vi "Martins HOT interface diag.vi"() -> ()   [LabVIEW 2012]
uses:
  Sub VIs/Trap cluster.ctl
  <vilib>/vision/Image Controls.llb/IMAQ Image.ctl
  Sub VIs/Get measurement coordinates.vi
  Sub VIs/Global variables.vi
  <vilib>/Utility/inputDevices.llb/closeKeyboard.vi
  <vilib>/Utility/inputDevices.llb/keyboardAcquire.vi
  <vilib>/Utility/file.llb/Write To Spreadsheet File (DBL).vi
  <vilib>/vision/driver/imaqhl.llb/IMAQ Grab Acquire.vi
  <vilib>/vision/driver/IMAQdx.llb/IMAQdx Grab.vi
  <vilib>/vision/driver/imaqll.llb/IMAQ Extract Buffer.vi
  Sub VIs/Get trap pos.vi
  <vilib>/Analysis/coordinate.llb/2D Cartesian Coordinate Shift.vi
  <vilib>/Analysis/coordinate.llb/2D Cartesian Coordinate Shift (Array).vi
  <vilib>/Analysis/coordinate.llb/2D Cartesian Coordinate Rotation.vi
  <vilib>/Analysis/coordinate.llb/2D Cartesian Coordinate Rotation (Scalar).vi
  <vilib>/vision/driver/NI_Vision_Acquisition_Software.lvlib
  <vilib>/vision/NI_Vision_Development_Module.lvlib
  <vilib>/Analysis/NI_AALPro.lvlib
panel:
  out "Using monitoring camera\nfor measurements":bool
  out "Measurement image":T1
  out "Monitoring image":T1
  in  "Apply Corrections":bool
  in  "View Licence":bool
  in  "ok":bool caption="Mark the center of \nthe spot using the \nzoom and the point\ntool, then click this \nbutton"
  in  "Stop program":bool
  in  "Updating trap cluster":bool
  out "Camera enabled":bool=TRUE
  out "SLM enabled":bool=TRUE
  in  "Hologram generation":cluster{"Method":i32, "Iterations":i32}={"Method"=1, "Iterations"=25} {"Method" items=["Lenses & Gratings (3D)", " Gerchberg-Saxton (3D)", "Gerchberg-Saxton FFT (2D)"]}
  in  "ROI":T2={"Global Rectangle"=[794, 414, 1159, 796], "Contours"=[{"Contour Type"=0, "ROI Type"=1, "Points"=[1158, 795]}, {"Contour Type"=0, "ROI Type"=1, "Points"=[898, 562]}, {"Contour Type"=0, "ROI Type"=1, "Points"=[794, 414]}]}
  out "Monitor image":T1(plugin-control)
  out "Waveform Graph":u32[](graph)
  out "max value":u32
  in  "reset":bool
  out "x/y":dbl
  in  "Outer bound":dbl=10.0
  in  "Inner bound":dbl=-10.0
  in  "stop \nsqueezing":bool
  in  "Squeeze":bool
  in  "Run meas calibration":bool
  in  "Display hologram\nand computed \nimage plane":bool
  in  "Run calibration":bool
  in  "Blank Button 2":bool
  in  "Blank Button":bool
  in  "subtract\nbackground":bool=TRUE
  in  "store \nbackground":bool
  in  "Coordinate mapping \n(Monitor to Measurement)":T3={"cZ"=1.0, "cY"=0.41527447, "cX"=-0.4158654, "sZ"=0.0, "sY"=-10.372314, "sX"=695.5264}
  in  "Transpose Measurement":bool
  out "Image\nsaturated":bool
  in  "Display ROIs":bool
  out "Lost Frames":u32=1
  in  "Display ROIs":bool
  out "Measurement image report":T4={"Mean Value"=58.96904, "Standard Variation"=5.129144, "Minimal Value"=35.0, "Maximal Value"=144.0, "Area (calibrated)"=65536.0, "Area (pixels)"=65536, "%"=100.0, "Calibration Valid"=TRUE} {"Mean Value" format="%.2f"; "%" format="%.2f"; "Area (calibrated)" format="%.2f"; "Maximal Value" format="%.2f"; "Minimal Value" format="%.2f"; "Standard Variation" format="%.2f"}
  in  "Save image path":path=path "E:/David/SLM characterization/Measured data/120420 - Trapping" caption="start path"
  in  "save image":bool
  in  "Edit trap cluster":bool
  in  "Display data":bool
  in  "Measure \nintensities":bool
  in  "Purge data":bool
  in  "ROI \nsize":dbl=24.0 min=2.0 step=2.0
  in  "Save data":bool
  in  "Record":bool
  in  "G":bool[](array[boolean])=[FALSE, FALSE, FALSE]
  out "Current trap pos":T5={"X (IMAQ)"=[1158.0, 898.0, 794.0], "Y (IMAQ)"=[795.0, 562.0, 414.0], "Z"=[0.0, 0.0, 0.0], "I"=[10.0, 10.0, 10.0], "Trap number"=[0, 1, 2], "ROI number"=[0, 1, 2], "Number of traps"=3, "Group"=[FALSE, FALSE, FALSE]}
  out "NI Vision error":errorcluster
  out "CUDA/SLM error":errorcluster
  in  "Cancel calibration":bool
  in  "Skip step if \ntimed out":bool
  in  "Display path":bool=TRUE
  out "Average step \ntime (ms)":dbl=14.596019900497513
  in  "Step \ntime \n(ms)":u32
  in  "Pause":bool
  in  "cancel path":bool
  out "Step \nskipped":bool
  in  "Path control":T6={"follow path"=FALSE, "Step \nlength"=0.2, "Arrive \nsimultaneously"=FALSE, "Synchronize traps"=FALSE, "Add current \npositions to path"=FALSE}
  in  "Create path":bool
  out "#":dbl[](array[numeric])=[0.0, 1.0, 2.0]
  in  "Group \nTraps":bool
  in  "Move \nHandle":bool
  in  "Coordinate mapping \n(IMAQ to SLM)":T3={"cZ"=1.0, "cY"=0.15274464, "cX"=0.15384616, "sZ"=-29.0, "sY"=-91.72315, "sX"=-108.5}
  in  "Transpose SLM":bool
  in  "I":dbl[](array[numeric])=[20.0, 20.0, 10.0]
  in  "Z":dbl[](array[numeric])=[0.0, 0.0, 0.0]
  # "Martin\nPersson 2011"
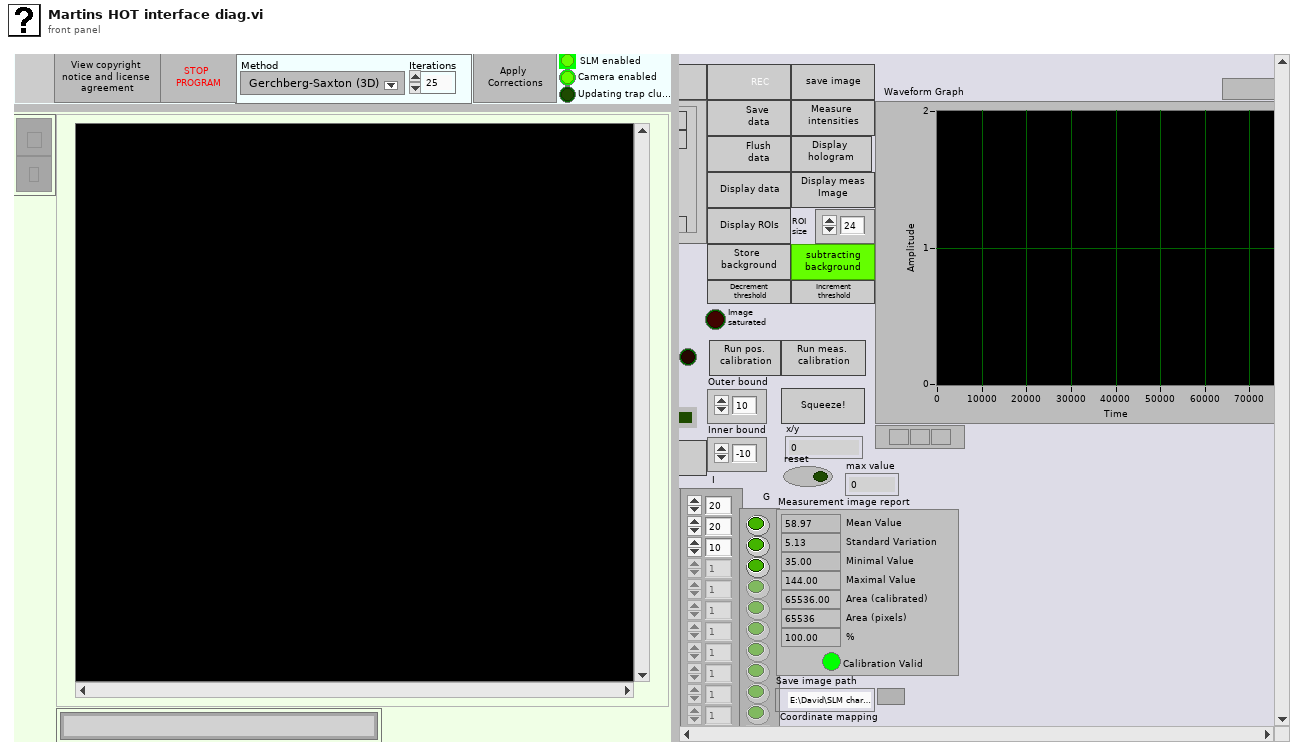
[diagram p1: front panel]
types:
  T1 = typedef "IMAQ Image.ctl" = refnum<image>
  T2 = cluster{"Global Rectangle":i32[], "Contours":cluster{"Contour Type":u32, "ROI Type":u32, "Points":i32[]}[]}
  T3 = cluster{"cZ":sgl, "cY":sgl, "cX":sgl, "sZ":sgl, "sY":sgl, "sX":sgl}
  T4 = cluster{"Mean Value":sgl, "Standard Variation":sgl, "Minimal Value":sgl, "Maximal Value":sgl, "Area (calibrated)":sgl, "Area (pixels)":u32, "%":sgl, "Calibration Valid":bool}
  T5 = typedef "Trap cluster.ctl" = cluster{"X (IMAQ)":sgl[], "Y (IMAQ)":sgl[], "Z":sgl[], "I":sgl[], "Trap number":i32[], "ROI number":i32[], "Number of traps":i32, "Group":bool[]}
  T6 = cluster{"follow path":bool, "Step \nlength":dbl, "Arrive \nsimultaneously":bool, "Synchronize traps":bool, "Add current \npositions to path":bool}
  T7 = cluster{"CentroidX":dbl[], "CentroidY":dbl[], "I":dbl[], "Acquired Buffer Number":u32}
  T8 = enum16{"IMAQ (Camera Link)", "IMAQ ring", "IMAQdx (firewire)", "No camera"}
  T9 = typedef "IMAQdx.ctl" = refnum<k21>
  T10 = cluster{"Camera type":enum16{"IMAQ (Camera Link)", "IMAQ ring", "IMAQdx (firewire)", "No camera"}, "IMAQ Session":refnum<k11>, "IMAQdx Session":T9, "Image":T1, "Image buffers":T1[], "Camera error":errorcluster}
  T11 = typedef "Image Type" = u32
  T12 = enum16{"Left Button", "Center Button", "Right Button", "Window Close"}
  T13 = typedef "ROI Descriptor" = cluster{"Global Rectangle":i32[], "Contours":cluster{"ID":enum32{"External", "Internal"}, "Type":u32, "Coordinates":i32[]}[]}
  T14 = enum16{"0", "1", "2", "3", "4", "5", "6", "7", "8", "9", "A", "B", "C", "D", "E", "F", "G", "H", "I", "J", "K", "L", "M", "N", "O", "P", "Q", "R", "S", "T", "U", "V", "W", "X", "Y", "Z", "F1", "F2", "F3", "F4", "F5", "F6", "F7", "F8", "F9", "F10", "F11", "F12", "F13", "F14", "F15", "ADD", "BACK", "BACKSLASH", "CAPITAL", "COMMA", "DECIMAL", "DELETE", "DIVIDE", "DOWN", "END", "EQUALS", "ESCAPE", "GRAVE (`)", "HOME", "INSERT", "LBRACKET", "LCONTROL", "LEFT", "L ALT", "LSHIFT", "LWIN", "MINUS", "MULTIPLY", "NEXT", "NUMLOCK", "NUMPAD_0", "NUMPAD_1", "NUMPAD_2", "NUMPAD_3", "NUMPAD_4", "NUMPAD_5", "NUMPAD_6", "NUMPAD_7", "NUMPAD_8", "NUMPAD_9", "PAUSE", "PERIOD", "PRIOR (PG UP)", "RBRACKET", "RCONTROL", "RETURN", "RIGHT", "R ALT", "RSHIFT", "RWIN", "SCROLL", "SEMICOLON", "SLASH", "SPACE", "SUBTRACT", "TAB", "UP", "ENTER (num pad)", "' (quote)"}[]
  T15 = cluster{"CentroidX":dbl[], "CentroidY":dbl[], "I":dbl[], "Acquired Buffer Number":u32}[]
  T16 = cluster{"Contour Type":u32, "ROI Type":u32, "Points":i32[]}[]
  T17 = cluster{"Contour Type":u32, "ROI Type":u32, "Points":i32[]}
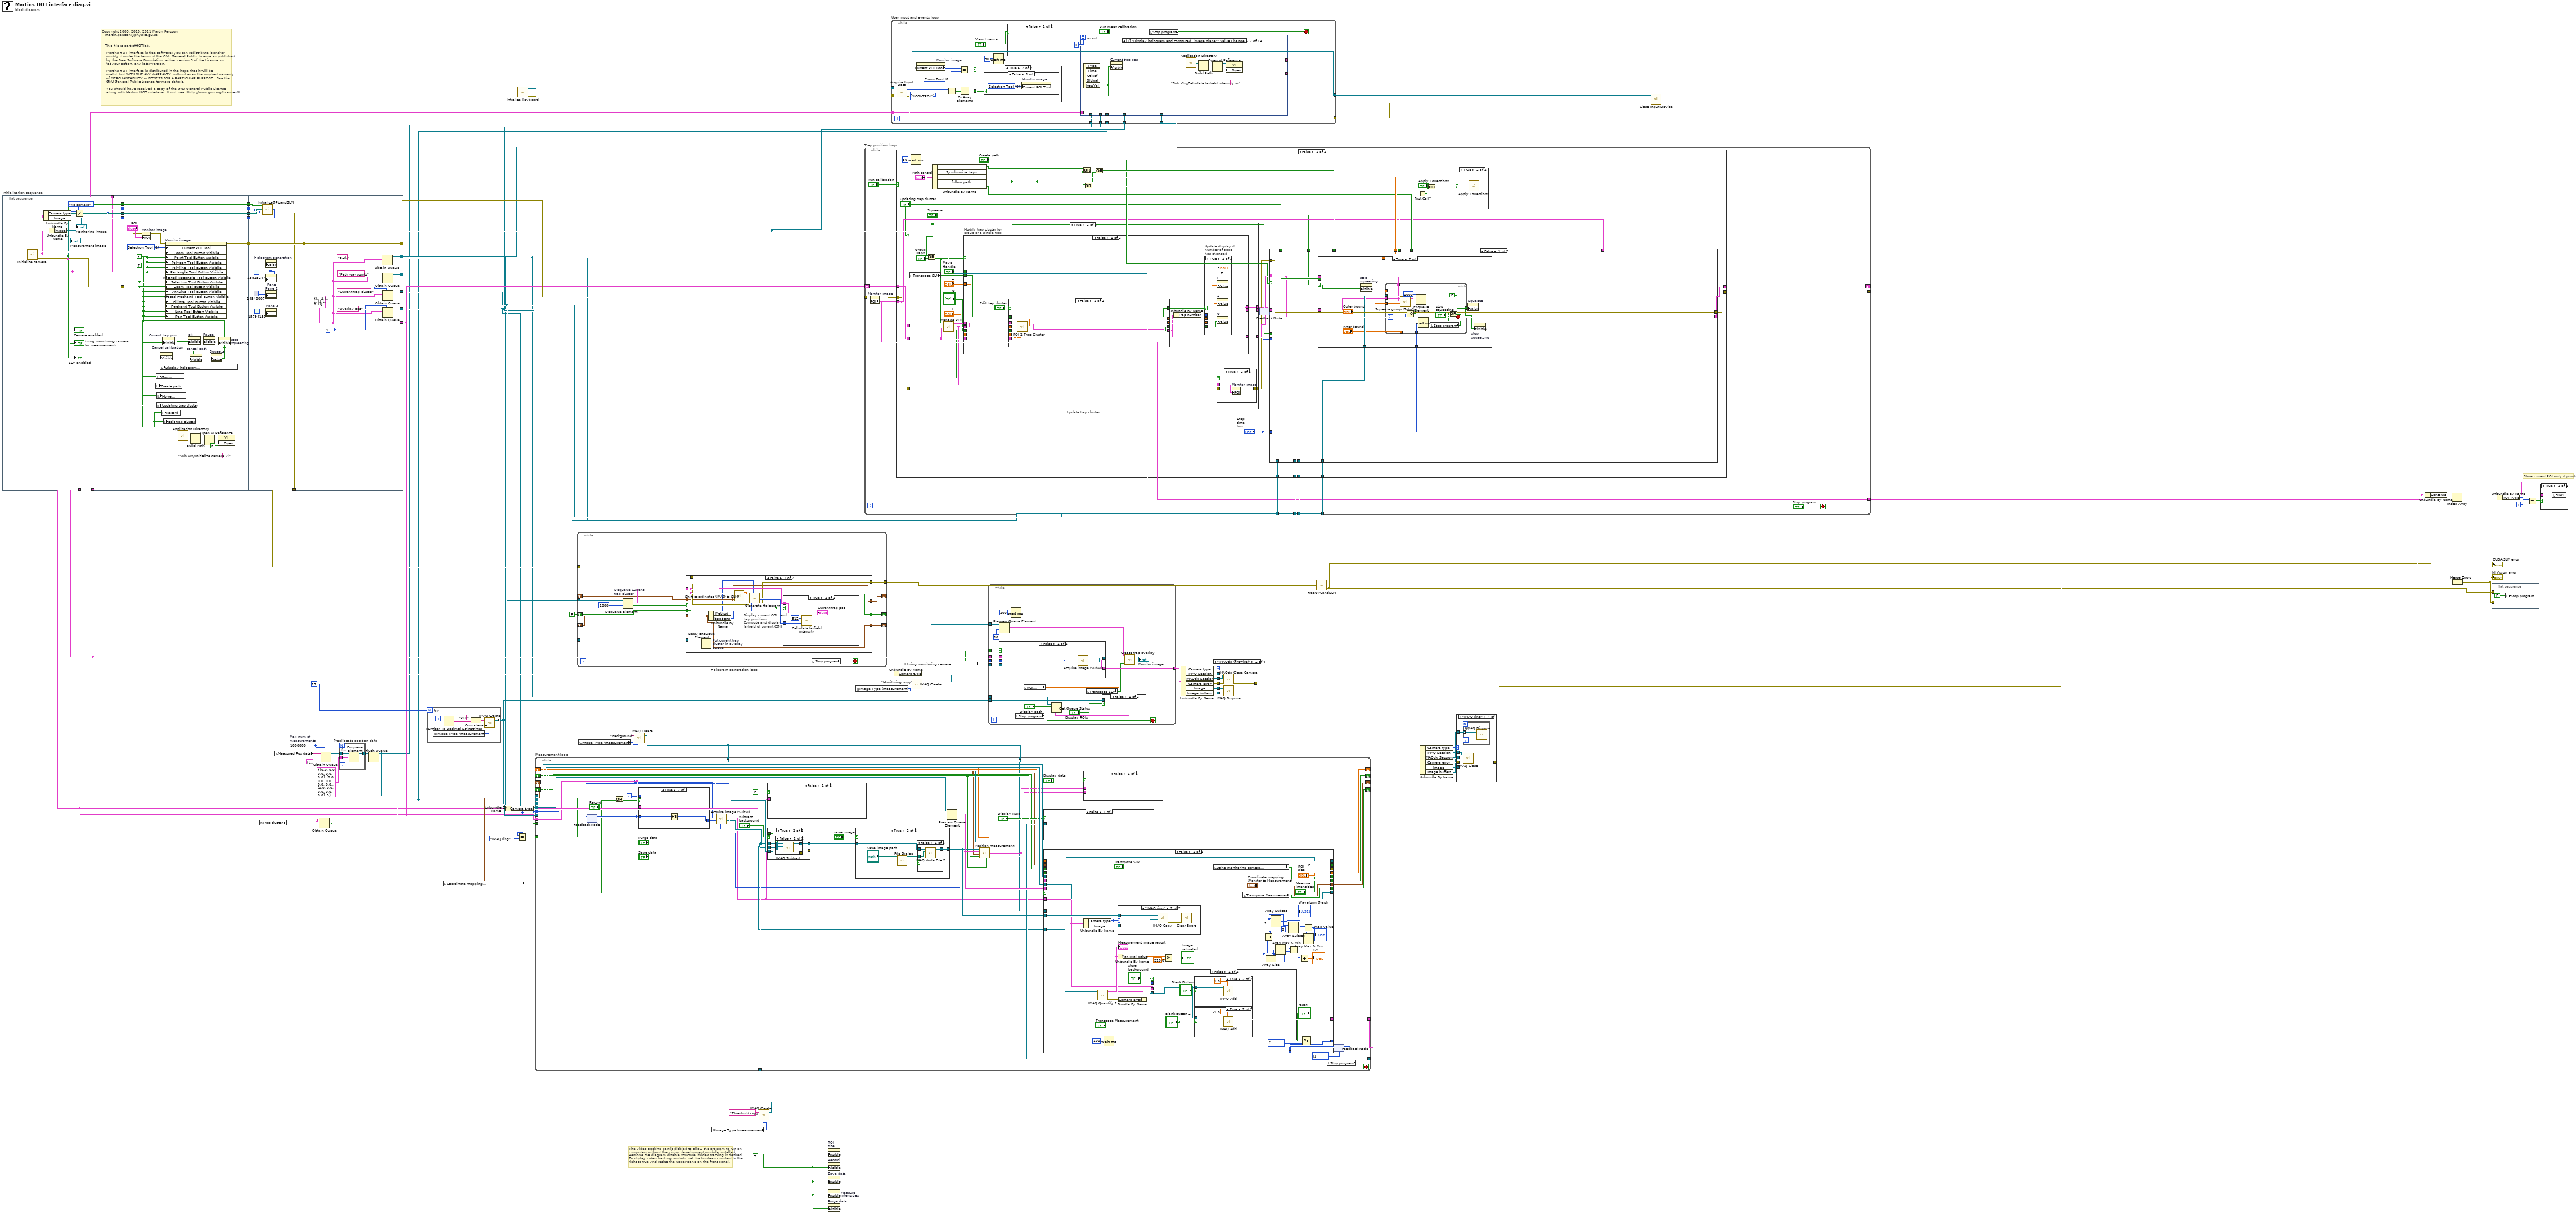
[diagram p0: block diagram]
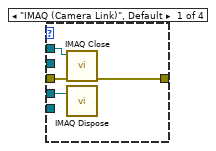
[diagram p2: hidden frame]
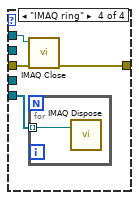
[diagram p4: hidden frame]
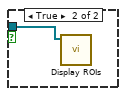
[diagram p5: hidden frame]
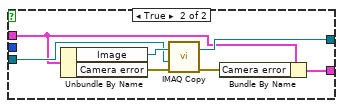
[diagram p6: hidden frame]
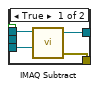
[diagram p8: hidden frame]
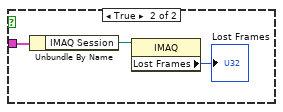
[diagram p9: hidden frame]
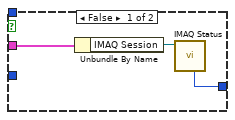
[diagram p10: hidden frame]
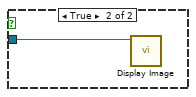
[diagram p11: hidden frame]
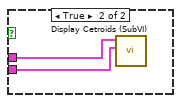
[diagram p12: hidden frame]
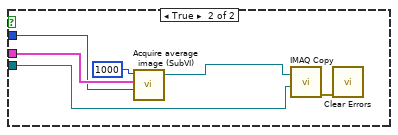
[diagram p17: hidden frame]
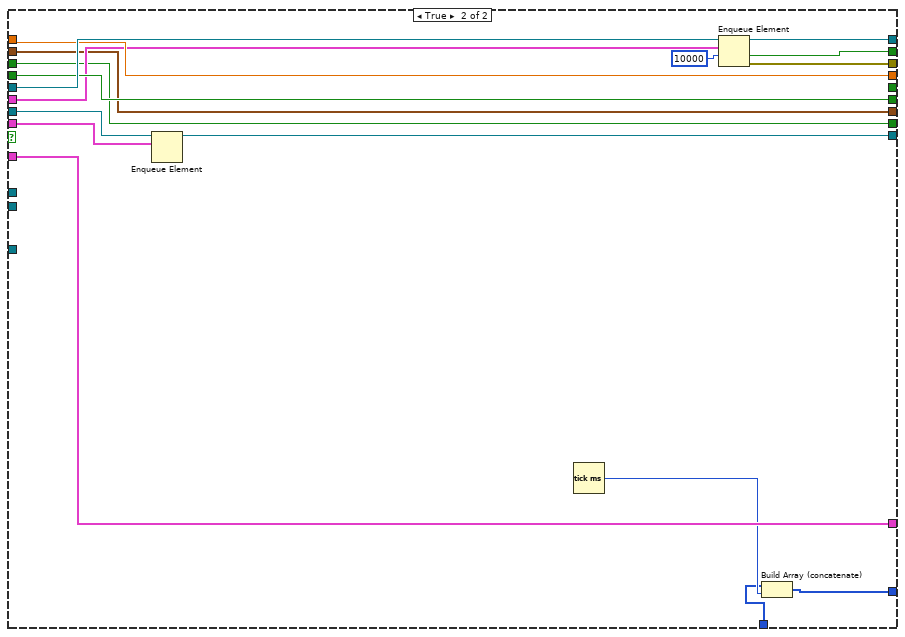
[diagram p19: hidden frame]
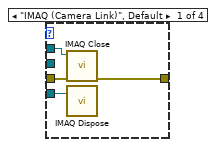
[diagram p20: hidden frame]
diagram:
  w1 = 1000000  # Max num of  measurements
  w77 = TRUE ("Visible")
  # "Copyright 2009, 2010, 2011 Martin Persson \n   martin.persson@physics.gu.se\n\n\n   This file is part ofHOTlab.\n\n    Martins HOT interface is free software: you can redistribute it and/or \n    modify it under the terms of the GNU General Public License as published \n    by the Free Software Foundation, either version 3 of the License, or\n    (at your option) any later version.\n\n    Martins HOT interface is distributed in the hope that it will be \n    useful, but WITHOUT ANY WARRANTY; without even the implied warranty\n    of MERCHANTABILITY or FITNESS FOR A PARTICULAR PURPOSE.  See the\n    GNU General Public License for more details.\n\n    You should have received a copy of the GNU General Public License\n    along with Martins HOT interface.  If not, see <http://www.gnu.org/licenses/>."
  # "Store current ROI only if points"
  # "The video tracking part is disbled to allow the program to run on\ncomputers without the vision development module installed. \nRemove the diagram disable structure ifvideo tracking is desired. \nTo diplay video tracking controls, set the boolean constant to the \nright to true And resize the upper pane on the front panel."
  n1 = flat-sequence "Initialization sequence" {
    tunnel: [w88] -> w63
    tunnel: [w92] -> w62
    tunnel: [w91] -> w61
    tunnel: [w90] -> w60
    tunnel: [w89] -> w59
    tunnel: [w83] -> w37
    tunnel: [w81] -> w9
    tunnel: [w81] -> w47
    tunnel: w63 -> [w105]
    tunnel: w62 -> [w103]
    tunnel: w61 -> [w108]
    tunnel: w60 -> [w107]
    tunnel: w59 -> [w106]
    tunnel: [w105] -> w55
    tunnel: [w100] -> w54
    tunnel: [w108] -> w52
    tunnel: [w107] -> w51
    tunnel: [w106] -> w50
    tunnel: w55 -> [w114]
    tunnel: w54 -> [w117]
    tunnel: [w117] -> w53
    tunnel: w52 -> [w115]
    tunnel: w51 -> [w116]
    tunnel: w50 -> [w113]
    tunnel: [w112] -> w49
    tunnel: [w128] -> w58
    tunnel: w53 -> [w128]
    tunnel: [w126] -> w24
    tunnel: [w124] -> w57
    tunnel: [w122] -> w48
    tunnel: [w121] -> w25
    tunnel: [w118] -> w56
    frame #0 {
      n2 = call "Initialize camera.vi"() -> ("Use monitoring camera\nfor measurements"=→"Using monitoring camera\nfor measurements":bool, "Vision error out"=w92:errorcluster, "CUDA device ID"=w90:i32, "TrueFrame out"=w91:i32, "Measurement camera cluster"=w81:T10, "LUT path out"=w89:path, "SLM enabled"=w88:bool, "Monitoring camera cluster"=w83:T10)  [unwired: 3 in]
      "SLM enabled" <- w88
      n3 = Unbundle By Name(w83) -> ("Camera type"=w85:T8, "Image"=→"Monitoring image":T1)
      n4 = Unbundle By Name(w81) -> ("Image"=→"Measurement image":T1)
      n5 = Not Equal?(x=w85, y=T8."No camera") -> (x != y?=→"Camera enabled":bool)
    }
    frame #1 {
      w99 = TRUE ("ROI Tool Buttons Visibile:Zoom Tool Button Visible")
      w98 = FALSE ("ROI Tool Buttons Visibile:Zoom Tool Button Visible")
      w102 = u32 0 items=["Zoom Tool"=8, "Selection Tool"=0, "Pan Tool"=9, "Point Tool"=1, "Line Tool"=2, "Rectangle Tool"=3, "Rotated Rectangle Tool"=12, "Polyline Tool"=10, "Polygon Tool"=5, "Freehand Tool"=11, "Closed Freehand Tool"=6, "Ellipse Tool"=4, "Annulus Tool"=7] ("Current ROI Tool")
      n6 = property on="Monitor image" class="ImageControl"(error in=w103, "ROI"="ROI") -> (error out=w101:errorcluster)  [unwired: 1 in, 1 out]
      n7 = local write "Create path"(w98) -> ()
      n8 = local write "Group \nTraps"(w98) -> ()
      n9 = local write "Move \nHandle"(w98) -> ()
      n10 = local write "Updating trap cluster"(w99) -> ()
      n11 = property on="Cancel calibration" class="Bool"("Visible"=w98) -> ()  [unwired: 2 in, 2 out]
      n12 = local write "Display hologram\nand computed \nimage plane"(w98) -> ()
      n13 = local write "Record"(w98) -> ()
      n14 = property on="Current trap pos" class="Clust (strict)"("Visible"=w98) -> ()  [unwired: 2 in, 2 out]
      n15 = local write "Edit trap cluster"(w98) -> ()
      n16 = property on="Monitor image" class="ImageControl"(error in=w101, "Current ROI Tool"=w102, "Zoom Tool Button Visibile"=w98, "Point Tool Button Visibile"=w98, "Polygon Tool Button Visibile"=w98, "Polyline Tool Button Visibile"=w98, "Rectangle Tool Button Visibile"=w98, "Rotated Rectangle Tool Button Visibile"=w98, "Selection Tool Button Visibile"=w99, "Zoom Tool Button Visibile"=w99, "Annulus Tool Button Visibile"=w98, "Closed Freehand Tool Button Visibile"=w98, "Ellipse Tool Button Visibile"=w98, "Freehand Tool Button Visibile"=w98, "Line Tool Button Visibile"=w98, "Pan Tool Button Visibile"=w98) -> (error out=w100:errorcluster)  [unwired: 1 in, 1 out]
      n17 = call <vilib>:"Application Directory.vi"() -> ("Application Directory"=w94:path)
      n18 = property on="ok" class="Bool"("Visible"=w98) -> ()  [unwired: 2 in, 2 out]
      n19 = property on="cancel path" class="Bool"("Visible"=w98) -> ()  [unwired: 2 in, 2 out]
      n20 = Build Path(base path=w94, name or relative path="Sub VIs\\Initialize camera.vi") -> (appended path=w97:path)
      n21 = property on="Pause" class="Bool (strict)"("Visible"=w98) -> ()  [unwired: 2 in, 2 out]
      n22 = Open VI Reference(vi path=w97) -> (vi reference=w96:refnum<vi>)  [unwired: 5 in, 1 out]
      n23 = property on="Squeeze" class="Bool (strict)"("Value"=w98) -> ()  [unwired: 2 in, 2 out]
      n24 = property class="VI"(reference=w96, "Front Panel.Open"=FALSE ("Front Panel Window:Open")) -> ()  [unwired: 1 in, 2 out]
      n25 = property on="stop \nsqueezing" class="Bool"("Visible"=w98) -> ()  [unwired: 2 in, 2 out]
    }
    frame #2 {
      w109 = u32 15925247 ("Pane Color")
      n26 = call "InitializeGPUandSLM.vi"("TrueFrame"=w115, "deviceId"=w116, "Path to LUT file"=w113, "SLM enabled"=w114) -> ("CUDA/SLM error"=w112:errorcluster)  [unwired: 1 out]
      n27 = property on="Hologram generation" class="Clust (strict)"("Color"=w109) -> ()  [unwired: 2 in, 2 out]
      n28 = property on="Pane" class="Pane"("PaneColor"=w109) -> ()  [unwired: 2 in, 2 out]
      n29 = property on="Pane 2" class="Pane"("PaneColor"=u32 14540007 ("Pane Color")) -> ()  [unwired: 2 in, 2 out]
      n30 = property on="Pane 3" class="Pane"("PaneColor"=u32 15794150 ("Pane Color")) -> ()  [unwired: 2 in, 2 out]
    }
    frame #3 {
      w118 = T5 {"X (IMAQ)"=[], "Y (IMAQ)"=[], "Z"=[], "I"=[], "Trap number"=[], "ROI number"=[], "Number of traps"=0, "Group"=[]} ("output cluster 2")
      w119 = 1 ("max queue size (-1, unlimited)")
      n31 = Obtain Queue(name (unnamed)="Path", element data type=w118) -> (queue out=w126:refnum<queue>)  [unwired: 3 in, 2 out]
      n32 = Obtain Queue(name (unnamed)="Path waypoints", element data type=w118) -> (queue out=w124:refnum<queue>)  [unwired: 3 in, 2 out]
      n33 = Obtain Queue(max queue size (-1, unlimited)=w119, name (unnamed)="Current trap cluster", element data type=w118) -> (queue out=w122:refnum<queue>)  [unwired: 2 in, 2 out]
      n34 = Obtain Queue(max queue size (-1, unlimited)=w119, name (unnamed)="Overlay pos", element data type=w118) -> (queue out=w121:refnum<queue>)  [unwired: 2 in, 2 out]
    }
  }
  n35 = global read "Global variables.vi" "Trap cluster"() -> (w13:string)
  n36 = global read "Global variables.vi" "Measured Pos data"() -> (w12:string)
  n37 = Obtain Queue(name (unnamed)=w13, element data type=w56) -> (queue out=w10:refnum<queue>, created new?=w11:bool)  [unwired: 3 in, 1 out]
  n38 = Obtain Queue(max queue size (-1, unlimited)=w1, name (unnamed)=w12, element data type=T7 {"CentroidX"=[], "CentroidY"=[], "I"=[], "Acquired Buffer Number"=0} ("Position data out")) -> (queue out=w5:refnum<queue>)  [unwired: 2 in, 2 out]
  n39 = for "Preallocate position data" {
    N: w1 -> [_]
    tunnel: w5 -> [w131]
    tunnel: T7 {"CentroidX"=[0.0, 0.0, 0.0, 0.0, 0.0], "CentroidY"=[0.0, 0.0, 0.0, 0.0, 0.0], "I"=[0.0, 0.0, 0.0, 0.0, 0.0], "Acquired Buffer Number"=5} ("Position data out") -> [w130]
    tunnel: [w129] -> w3
    n40 = Enqueue Element(queue=w131, element=w130) -> (queue out=w129:refnum<queue>)  [unwired: 2 in, 2 out]
  }
  n41 = Flush Queue(queue=w3) -> (queue out=w2:refnum<queue>)  [unwired: 1 in, 2 out]
  n42 = for {
    N: 25 -> [_]
    tunnel: [w137] -> w23 mode=indexing
    i -> [w134]
    n43 = global read "Global variables.vi" "Image Type (measurement)"() -> (w132:T11)
    n44 = Number To Decimal String(number=w134) -> (decimal integer string=w133:string)  [unwired: 1 in]
    n45 = Concatenate Strings("ROI" ("Image Name"), w133) -> (w135:string)
    n46 = call "IMAQ Create"("Image Name"=w135, "Image Type"=w132) -> ("New Image"=w137:T1)  [unwired: 3 in, 1 out]
  }
  n47 = local read "Coordinate mapping \n(Monitor to Measurement)"() -> (w18:T3)
  n48 = Unbundle By Name(w9) -> ("Camera type"=w7:T8)
  n49 = Not Equal?(x=w7, y=T8."IMAQ ring") -> (x != y?=w8:bool)
  n50 = call <vilib>:"Intialize Keyboard.vi"() -> ("error out"=w65:errorcluster, "device ID"=w79:refnum<k1>)  [unwired: 1 in, 9 out]
  n51 = while "Hologram generation loop" {
    tunnel: w48 -> [w149]
    tunnel: w25 -> [w147]
    tunnel: w49 -> [w146]
    tunnel: [w145] -> w46
    shift-right: [w144] -> _
    shift-left: _ -> [w143]
    shift-right: [w142] -> _
    shift-left: _ -> [w141]
    shift-right: [w140] -> _
    shift-left: FALSE ("Display hologram\nand computed \nimage plane") -> [w139]
    stop <- w150 stop-if-true
    n52 = Dequeue Element "Dequeue Current \ntrap cluster"(queue=w149, timeout in ms (-1)=1000) -> (element=w148:T5, timed out?=w138:bool)  [unwired: 1 in, 2 out]
    n53 = case shown="False" w138 {
      tunnel: w143 -> [w156 _]
      tunnel: w148 -> [w160 _]
      tunnel: w147 -> [w159 _]
      tunnel: w146 -> [w158 w172]
      tunnel: [w157 w172] -> w145
      tunnel: [w156 "Coordinate mapping \n(IMAQ to SLM)"] -> w144
      tunnel: [w153 "Hologram generation"] -> w142
      tunnel: w141 -> [w153 _]
      tunnel: [w152 "Display hologram\nand computed \nimage plane"] -> w140
      tunnel: w139 -> [w152 _]
      frame False {
        n54 = Lossy Enqueue Element "Put current trap \ncluster in overlay \nqueue"(queue=w159, element=w160) -> ()  [unwired: 1 in, 4 out]
        n55 = Unbundle By Name(w153) -> ("Method"=w155:i32, "Iterations"=w154:i32)
        n56 = call "Shift coordinates (IMAQ to SLM).vi"("Trap cluster"=w160, "Coordinate mapping \n(IMAQ to SLM)"=w156) -> ("X (SLM)"=w161:sgl[], "Y (SLM)"=w164:sgl[], "Intensities"=w162:sgl[], "Z (SLM)"=w163:sgl[])  [unwired: 1 in, 1 out]
        n57 = call "Generate Hologram.vi"("x"=w161, "y"=w164, "z"=w163, "spot_intensities"=w162, "CUDA/SLM error in"=w158, "N_iterations"=w154, "method"=w155) -> ("CGH out"=w165:u8[][], "CUDA/SLM error out"=w157:errorcluster)  [unwired: 17 in, 2 out]
        n58 = case "Display current CGH and trap positions.\nCompute and display farfield of current CGH" shown="True" w152 {
          tunnel: w165 -> [_ w168]
          tunnel: w160 -> [_ w167]
          frame False {
          }
          frame True {
            n59 = call "Calculate farfield intensity.vi"("h_pSLM"=w168, "SLMsize"=512 ("Numeric")) -> ()  [unwired: 1 out]
            "Current trap pos" <- w167
          }
        }
      }
      frame True {
      }
    }
    n60 = local read "Stop program"() -> (w150:bool)
  }
  n61 = global read "Global variables.vi" "Image Type (measurement)"() -> (w16:T11)
  n62 = call "IMAQ Create"("Image Name"="Background", "Image Type"=w16) -> ("New Image"=w14:T1)  [unwired: 3 in, 1 out]
  n63 = global read "Global variables.vi" "Image Type (measurement)"() -> (w20:T11)
  n64 = call "IMAQ Create"("Image Name"="Threshold copy", "Image Type"=w20) -> ("New Image"=w22:T1)  [unwired: 3 in, 1 out]
  n65 = while "Measurement loop" {
    tunnel: w23 -> [w203]
    tunnel: w2 -> [w212]
    shift-right: [w211] -> _
    shift-left: _ -> [w201]
    tunnel: w10 -> [w210]
    shift-right: [w209] -> _
    shift-left: _ -> [w202]
    tunnel: [w204] -> _
    tunnel: w9 -> [w194]
    tunnel: w25 -> [w206]
    tunnel: w24 -> [_]
    tunnel: [w207] -> w40
    tunnel: w7 -> [w180]
    tunnel: w22 -> [w184]
    shift-right: [w197] -> _
    shift-left: w18 -> [w196]
    shift-right: [w190] -> _
    shift-left: _ -> [w189]
    tunnel: w14 -> [w188]
    tunnel: w14 -> [w186]
    tunnel: w11 -> [_]
    tunnel: w8 -> [w178]
    i -> [w192]
    stop <- w213 stop-if-true
    n66 = feedback #1() -> (w182:u32)  [unwired: 1 in]
    n67 = Or(x=w178, y="Record") -> (x .or. y?=w179:bool)
    n68 = case shown="True" w179 {
      tunnel: w194 -> [w235 _]
      tunnel: [w233 w236] -> w193
      tunnel: w192 -> [_ _]
      tunnel: w182 -> [_ w237]
      frame False {
        n69 = Unbundle By Name(w235) -> ("IMAQ Session"=w234:refnum<k11>)
        n70 = call <vilib>:"IMAQ Status.vi"("IMAQ Session In"=w234) -> ("Last Valid Buffer Number"=w233:i32)  [unwired: 6 in, 4 out]
      }
      frame True {
        n71 = Increment(x=w237) -> (x+1=w236:u32)
      }
    }
    n72 = call "Acquire image (SubVI).vi"("Buffer number"=w193, "Camera type"=w180, "Measurement camera \ncluster in"=w194) -> ("Image Out"=w181:T1, "Measurement camera cluster out"=w177:T10, "Buffer Number Out"=w183:u32)  [unwired: 6 in]
    n73 = feedback-in #1(w183) -> ()
    n74 = case shown="False" FALSE {
      tunnel: w177 -> [_ w230]
      frame False {
      }
      frame True {
        n75 = Unbundle By Name(w230) -> ("IMAQ Session"=w232:refnum<k11>)
        n76 = property class="IMAQ"(reference=w232) -> ("Lost Frames"=→"Lost Frames":u32)  [unwired: 1 in, 2 out]
      }
    }
    n77 = case shown="True" "subtract\nbackground" {
      tunnel: [w214 w220] -> w187
      tunnel: w181 -> [w214 w219]
      tunnel: w186 -> [_ w218]
      tunnel: [_ w217] -> _
      tunnel: w184 -> [_ w215]
      tunnel: "Record" -> [_ w216]
      frame False {
      }
      frame True {
        n78 = case shown="False" w216 {
          tunnel: [w224 w229] -> w220
          tunnel: w219 -> [w223 w228]
          tunnel: w218 -> [w222 w227]
          tunnel: [w221 w226] -> w217
          tunnel: w215 -> [_ w225]
          frame True {
            n79 = call "IMAQ Subtract"("Image Src A"=w223, "Image Src B"=w222) -> ("Image Dst Out"=w224:T1, "error out"=w221:errorcluster)  [unwired: 5 in]
          }
          frame False {
            n80 = call "IMAQ Subtract"("Image Src A"=w228, "Image Dst"=w225, "Image Src B"=w227) -> ("Image Dst Out"=w229:T1, "error out"=w226:errorcluster)  [unwired: 4 in]
          }
        }
      }
    }
    n81 = case shown="True" "save image" {
      tunnel: w187 -> [w241 w246]
      tunnel: [w241 w245] -> w204
      frame False {
      }
      frame True {
        n82 = call "File Dialog"("start path"="Save image path") -> ("selected path"=w244:path, "cancelled"=w243:bool)  [unwired: 11 in, 2 out]
        n83 = case shown="False" w243 {
          tunnel: w246 -> [w249 w250]
          tunnel: [w248 w250] -> w245
          tunnel: w244 -> [w247 _]
          frame False {
            n84 = call-poly "IMAQ Write File 2"("File Path"=w247, "Image"=w249) -> ("Image Out (duplicate)"=w248:T1)  [unwired: 8 in, 1 out]
          }
          frame True {
          }
        }
      }
    }
    n85 = Preview Queue Element(queue=w206) -> (element=w205:T5)  [unwired: 2 in, 3 out]
    n86 = call "Position measurement.vi"("Measure \nintensities"=w202, "ROI size"=w201, "Acquired Buffer Number"=w182, "Switch xy"=w189, "Coordinate mapping \n(Monitor to Measurement)"=w196, "ROIs"=w203, "Trap positions"=w205, "Image"=w204) -> ("Target coordinates"=w195:cluster{"X target":sgl[], "Y target":sgl[]}, "Position data out"=w199:T7)  [unwired: 1 in]
    n87 = case shown="False" "Display ROIs" {
      tunnel: w204 -> [_ w238]
      frame False {
      }
      frame True {
        n88 = call "Display Image.vi"("Image 2"=w238) -> ()  [unwired: 11 in]
      }
    }
    n89 = case shown="False" "Display data" {
      tunnel: w199 -> [_ w240]
      tunnel: w195 -> [_ w239]
      frame False {
      }
      frame True {
        n90 = call "Display Cetroids (SubVI).vi"("Target coordinates"=w239, "Measurement data"=w240) -> ()  [unwired: 7 in, 3 out]
      }
    }
    n91 = local read "Stop program"() -> (w213:bool)
    n92 = feedback #2(u32[] []) -> (w175:u32[])
    n93 = case shown="False" "Record" {
      tunnel: w212 -> [w288 w321]
      tunnel: [w288 w320] -> _
      tunnel: [_ w319] -> _
      tunnel: ["ROI \nsize" w318] -> w211
      tunnel: w201 -> [_ w318]
      tunnel: w210 -> [w287 w317]
      tunnel: [w287 w316] -> _
      tunnel: ["Measure \nintensities" w315] -> w209
      tunnel: w202 -> [_ w315]
      tunnel: [FALSE ("timed out?") w313] -> _
      tunnel: w204 -> [w271 _]
      tunnel: w177 -> [w269 w312]
      tunnel: [w281 w312] -> w207
      tunnel: w205 -> [_ w311]
      tunnel: w199 -> [_ w310]
      tunnel: ["Coordinate mapping \n(Monitor to Measurement)" w309] -> w197
      tunnel: w196 -> [_ w309]
      tunnel: [w275 _] -> _
      tunnel: [w273 w308] -> w190
      tunnel: w189 -> [_ w308]
      tunnel: w188 -> [w270 _]
      tunnel: w181 -> [w267 _]
      tunnel: [w266 w307] -> w176
      tunnel: w175 -> [w255 w305]
      frame False {
        n94 = Unbundle By Name(w269) -> ("Camera type"=w268:T8, "Image"=w274:T1)
        n95 = call "IMAQ Quantify 2"("Image"=w267) -> ("error out"=w282:errorcluster, "Global Report"=w280:T4)  [unwired: 8 in, 1 out]
        "Measurement image report" <- w280
        n96 = Wait (ms)(milliseconds to wait=u32 100) -> ()  [unwired: 1 out]
        n97 = case shown="\"IMAQ ring\"" w268 {
          tunnel: w271 -> [_ w304]
          tunnel: w274 -> [_ w303]
          frame "IMAQ (Camera Link)", Default {
          }
          frame "IMAQ ring" {
            n98 = call "IMAQ Copy"("Image Dst"=w303, "Image Src"=w304) -> ("error out"=w302:errorcluster)  [unwired: 4 in, 1 out]
            n99 = call <vilib>:"Clear Errors.vi"("error in (no error)"=w302) -> ()  [unwired: 6 in, 1 out]
          }
        }
        n100 = Unbundle By Name(w280) -> ("Maximal Value"=w279:sgl)
        n101 = Bundle By Name(cluster=w269, "Camera error"=w282) -> (w281:T10)
        n102 = case shown="False" "store \nbackground" {
          tunnel: w270 -> [w291 w300]
          tunnel: w269 -> [_ w299]
          tunnel: w268 -> [_ w298]
          frame False {
            n103 = case shown="True" "Blank Button" {
              tunnel: w291 -> [_ w295]
              frame False {
              }
              frame True {
                n104 = call "IMAQ Add"("Image Src A"=w295, "Constant"=sgl 1.0) -> ()  [unwired: 5 in, 2 out]
              }
            }
            n105 = case shown="True" "Blank Button 2" {
              tunnel: w291 -> [_ w293]
              frame False {
              }
              frame True {
                n106 = call "IMAQ Add"("Image Src A"=w293, "Constant"=sgl -1.0) -> ()  [unwired: 5 in, 2 out]
              }
            }
          }
          frame True {
            n107 = call "Acquire average image (SubVI).vi"("Camera type"=w298, "Measurement camera cluster in"=w299, "averaging time (ms)"=1000) -> ("Refnum out"=w296:T1)  [unwired: 8 in]
            n108 = call "IMAQ Copy"("Image Dst"=w300, "Image Src"=w296) -> ("error out"=w301:errorcluster)  [unwired: 4 in, 1 out]
            n109 = call <vilib>:"Clear Errors.vi"("error in (no error)"=w301) -> ()  [unwired: 6 in, 1 out]
          }
        }
        n110 = Greater Or Equal?(x=w279, y=sgl 210.0) -> (x >= y?=→"Image\nsaturated":bool)
        n111 = local read "Using monitoring camera\nfor measurements"() -> (w275:bool)
        n112 = local read "Transpose Measurement"() -> (w273:bool)
        n113 = Array Size(array=w255) -> (size(s)=w259:i32)
        n114 = Decrement(x=w259) -> (x-1=w257:i32)
        n115 = Array Subset(array=w255, index=1, length=w257) -> (w254:u32[])
        n116 = Array Max & Min(array=w255) -> (max value=w262:u32, min value=w261:u32)  [unwired: 2 out]
        n117 = Array Subset(array=w255, index=0, length=w257) -> (w253:u32[])
        n118 = Subtract(x=w262, y=w261) -> (x-y=w260:u32)
        n119 = Divide(x=w259, y=w260) -> (x/y=→"x/y":dbl)
        n120 = Select(t=u32[] [], s="reset", f=w255) -> (s? t:f=w266:u32[])
        n121 = Subtract(x=w254, y=w253) -> (x-y=w251:u32[])
        "Waveform Graph" <- w251
        n122 = Array Max & Min(array=w251) -> (max value=→"max value":u32)  [unwired: 3 out]
      }
      frame True {
        n123 = Enqueue Element(queue=w317, element=w311) -> (queue out=w316:refnum<queue>)  [unwired: 2 in, 2 out]
        n124 = Tick Count (ms)() -> (millisecond timer value=w306:u32)
        n125 = Enqueue Element(queue=w321, element=w310, timeout in ms (-1)=10000) -> (queue out=w320:refnum<queue>, timed out?=w313:bool, error out=w319:errorcluster)  [unwired: 1 in]
        n126 = Build Array (concatenate)(w305, w306) -> (w307:u32[])
      }
    }
    n127 = feedback-in #2(w176) -> ()
  }
  n128 = property on="ROI \nsize" class="DigNum (strict)"("Visible"=w77) -> ()  [unwired: 2 in, 2 out]
  n129 = property on="Record" class="Bool (strict)"("Visible"=w77) -> ()  [unwired: 2 in, 2 out]
  n130 = property on="Save data" class="Bool"("Visible"=w77) -> ()  [unwired: 2 in, 2 out]
  n131 = property on="Measure \nintensities" class="Bool (strict)"("Visible"=w77) -> ()  [unwired: 2 in, 2 out]
  n132 = property on="Purge data" class="Bool"("Visible"=w77) -> ()  [unwired: 2 in, 2 out]
  n133 = global read "Global variables.vi" "Image Type (measurement)"() -> (w19:T11)
  n134 = while "Trap position loop" {
    tunnel: w57 -> [w333]
    tunnel: w24 -> [w330]
    shift-right: [w332] -> _
    shift-left: w56 -> [w325]
    tunnel: w48 -> [w331]
    tunnel: w25 -> [w328]
    tunnel: [w327] -> w71
    tunnel: w58 -> [w324]
    tunnel: [w322] -> w69
    stop <- "Stop program" stop-if-true
    n135 = property on="Monitor image" class="ImageControl"(error in=w324) -> (error out=w323:errorcluster, "ROI"=w327:T2)  [unwired: 1 in, 1 out]
    n136 = case shown="False" "Run calibration" {
      selector: "Run calibration" -> [_ w581]
      tunnel: w333 -> [w363 _]
      tunnel: w325 -> [w362 w580]
      tunnel: [w342 w580] -> w332
      tunnel: w331 -> [w352 w589]
      tunnel: w330 -> [w351 _]
      tunnel: w328 -> [w348 _]
      tunnel: w327 -> [w347 w588]
      tunnel: w323 -> [w346 w585]
      tunnel: [w344 w582] -> w322
      frame False {
        n137 = Wait (ms)(milliseconds to wait=u32 50) -> ()  [unwired: 1 out]
        n138 = Unbundle By Name("Path control") -> ("Add current \npositions to path"=w349:bool, "Synchronize traps"=w357:bool, "Step \nlength"=w360:dbl, "follow path"=w336:bool, "Arrive \nsimultaneously"=w359:bool)
        n139 = Or(x=w349, y=w357) -> (x .or. y?=w358:bool)
        n140 = Or(x=w357, y=w336) -> (x .or. y?=w355:bool)
        n141 = Or(x=w358, y=w336) -> (x .or. y?=w356:bool)
        n142 = feedback #3() -> (w334:T2)  [unwired: 1 in]
        n143 = case "Update trap cluster" shown="True" "Updating trap cluster" {
          tunnel: w362 -> [w366 w384]
          tunnel: [w366 w377] -> w353
          tunnel: w347 -> [_ w375]
          tunnel: w346 -> [w365 w374]
          tunnel: [w365 w373] -> w345
          tunnel: "Squeeze" -> [_ w369]
          tunnel: [w364 w368] -> w335
          tunnel: w334 -> [w364 w367]
          frame False {
          }
          frame True {
            n144 = local read "Transpose SLM"() -> (w383:bool)
            n145 = Or(x=w369, y="Group \nTraps") -> (x .or. y?=w370:bool)
            n146 = call "Manage ROI.vi"("Switch X/Y"=w383, "Trap cluster in"=w384, "ROI in"=w375, "Group traps"=w370) -> ("Replace ROI"=w371:bool, "ROI out"=w376:T2, "Previous ROI out"=w382:T2)
            n147 = case "Modify trap cluster for \ngroup or a single trap" shown="False" w370 {
              tunnel: [w395 w435] -> w377
              tunnel: w376 -> [w402 w429]
              tunnel: w384 -> [w401 w437]
              tunnel: w382 -> [_ w436]
              tunnel: "Z" -> [w400 w434]
              tunnel: "Move \nHandle" -> [_ w433]
              tunnel: w383 -> [w399 w432]
              tunnel: "I" -> [w397 w431]
              tunnel: "G" -> [w392 w430]
              tunnel: [w389 w429] -> w368
              tunnel: w367 -> [w389 _]
              frame False {
                n148 = case shown="False" "Edit trap cluster" {
                  tunnel: w402 -> [w413 w416]
                  tunnel: w401 -> [w412 w424]
                  tunnel: w400 -> [w411 _]
                  tunnel: w399 -> [w410 _]
                  tunnel: [w409 w423] -> w398
                  tunnel: w397 -> [w408 _]
                  tunnel: [w407 w422] -> w396
                  tunnel: [w406 w418] -> w395
                  tunnel: [w405 TRUE ("Update display")] -> w393
                  tunnel: w392 -> [w404 _]
                  tunnel: [w403 w420] -> w391
                  frame False {
                    n149 = call "ROI 2 Trap Cluster.vi"("Amplitudes"=w408, "Switch X/Y"=w410, "Group"=w404, "Trap Cluster in"=w412, "Z"=w411, "ROI"=w413) -> ("Group out"=w403:bool[], "Z out"=w409:dbl[], "Amplitudes out"=w407:dbl[], "Trap Cluster Out"=w406:T5, "Update display"=w405:bool)
                  }
                  frame True {
                    n150 = local read "Coordinate mapping \n(IMAQ to SLM)"() -> (w415:T3)
                    n151 = call "Edit trap cluster.vi"("Coordinate mapping \n(IMAQ to SLM)"=w415, "trap cluster in"=w424) -> ("SubVI closed"=w419:bool, "Trap cluster out"=w418:T5)
                    n152 = Not(x=w419) -> (.not. x?=w414:bool)
                    n153 = call "Trap cluster 2 ROI.vi"("Trap cluster"=w418, "ROI in"=w416) -> ("ROI out"=w417:T2)  [unwired: 1 in]
                    n154 = property on="Monitor image" class="ImageControl"("ROI"=w417) -> ()  [unwired: 2 in, 2 out]
                    n155 = local write "Edit trap cluster"(w414) -> ()
                    n156 = Unbundle By Name(w418) -> ("Z"=w423:sgl[], "I"=w422:sgl[], "Group"=w420:bool[])
                  }
                }
                n157 = Unbundle By Name(w395) -> ("Trap number"=w394:i32[])
                n158 = case "Update display if\nnumber of traps \nhas changed" shown="True" w393 {
                  tunnel: w398 -> [_ w428]
                  tunnel: w396 -> [_ w427]
                  tunnel: w394 -> [_ w426]
                  tunnel: w391 -> [_ w425]
                  frame False {
                  }
                  frame True {
                    n159 = property on="I" class="Arr (strict)"("Value"=w427) -> ()  [unwired: 2 in, 2 out]
                    n160 = property on="Z" class="Arr (strict)"("Value"=w428) -> ()  [unwired: 2 in, 2 out]
                    n161 = property on="G" class="Arr (strict)"("Value"=w425) -> ()  [unwired: 2 in, 2 out]
                    "#" <- w426
                  }
                }
              }
              frame True {
                n162 = call "Move group.vi"("New handle position in"=w429, "Trap cluster in"=w437, "Previous handle position in"=w436, "Amplitudes"=w431, "Group"=w430, "Switch X/Y"=w432, "Move handle"=w433, "Z"=w434) -> ("Trap cluster out"=w435:T5)
              }
            }
            n163 = case shown="True" w371 {
              tunnel: w376 -> [_ w388]
              tunnel: w374 -> [w385 w387]
              tunnel: [w385 w386] -> w373
              frame False {
              }
              frame True {
                n164 = property on="Monitor image" class="ImageControl"(error in=w387, "ROI"=w388) -> (error out=w386:errorcluster)  [unwired: 1 in, 1 out]
              }
            }
          }
        }
        n165 = feedback-in #3(w335) -> ()
        n166 = case shown="False" "Create path" {
          tunnel: w363 -> [_ w482]
          tunnel: w353 -> [w442 w476]
          tunnel: w360 -> [w438 w491]
          tunnel: w351 -> [_ w486]
          tunnel: w359 -> [_ w490]
          tunnel: w356 -> [_ w489]
          tunnel: w355 -> [_ w488]
          tunnel: w336 -> [_ w487]
          tunnel: w352 -> [w445 w483]
          tunnel: w348 -> [_ w481]
          tunnel: w347 -> [_ w480]
          tunnel: w345 -> [w444 w479]
          tunnel: [w444 w478] -> w344
          tunnel: "Updating trap cluster" -> [w443 _]
          tunnel: [w442 w477] -> w342
          tunnel: "Squeeze" -> [w441 _]
          tunnel: w334 -> [w440 _]
          tunnel: "Step \ntime \n(ms)" -> [_ w475]
          tunnel: "Step \ntime \n(ms)" -> [w439 _]
          frame False {
            n167 = case shown="True" w441 {
              selector: w441 -> [_ w452]
              tunnel: w445 -> [w448 w459]
              tunnel: w443 -> [w447 _]
              tunnel: w442 -> [w446 w458]
              tunnel: w440 -> [_ w457]
              tunnel: w439 -> [_ w454]
              tunnel: w438 -> [_ w453]
              frame False {
                n168 = case shown="True" w447 {
                  tunnel: w446 -> [_ w450]
                  tunnel: w448 -> [_ w449]
                  frame False {
                  }
                  frame True {
                    n169 = Lossy Enqueue Element(queue=w449, element=w450) -> ()  [unwired: 1 in, 4 out]
                  }
                }
              }
              frame True {
                n170 = property on="stop \nsqueezing" class="Bool"("Visible"=w452) -> ()  [unwired: 2 in, 2 out]
                n171 = while {
                  tunnel: w459 -> [w474]
                  tunnel: w458 -> [w473]
                  tunnel: w457 -> [w472]
                  tunnel: "Outer bound" -> [w471]
                  tunnel: "Inner bound" -> [w470]
                  tunnel: w453 -> [w469]
                  tunnel: [FALSE ("Squeeze")] -> w451
                  tunnel: w454 -> [w462]
                  i -> [w466]
                  stop <- w461 stop-if-true
                  n172 = Equal To 0?(x=w466) -> (x = 0?=w465:bool)
                  n173 = call "Squeeze group (SubVI).vi"("reset"=w465, "Step length"=w469, "Inner bound"=w470, "Outer bound"=w471, "Trap cluster in"=w473, "ROI in"=w472) -> ("output cluster"=w468:T5)  [unwired: 5 in]
                  n174 = Enqueue Element(queue=w474, element=w468, timeout in ms (-1)=1000) -> ()  [unwired: 1 in, 3 out]
                  n175 = Wait (ms)(milliseconds to wait=w462) -> ()  [unwired: 1 out]
                  n176 = local read "Stop program"() -> (w460:bool)
                  n177 = Or(x=w460, y="stop \nsqueezing") -> (x .or. y?=w461:bool)
                }
                n178 = property on="Squeeze" class="Bool (strict)"("Value"=w451) -> ()  [unwired: 2 in, 2 out]
                n179 = property on="stop \nsqueezing" class="Bool"("Visible"=w451) -> ()  [unwired: 2 in, 2 out]
              }
            }
          }
          frame True {
            n180 = Lossy Enqueue Element "Enqueue\noverlay pos"(queue=w481, element=w476) -> ()  [unwired: 1 in, 4 out]
            n181 = case "Add wpt" shown="True" w489 {
              tunnel: w476 -> [_ w570]
              tunnel: w482 -> [w567 w571]
              tunnel: [w567 w568] -> w492
              tunnel: [_ w569] -> w484
              frame False {
              }
              frame True {
                n182 = Enqueue Element "Enqueue path\n waypts"(queue=w571, element=w570) -> (queue out=w568:refnum<queue>, error out=w569:errorcluster)  [unwired: 2 in, 1 out]
              }
            }
            n183 = case "Compute path" shown="True" w488 {
              tunnel: w492 -> [_ w578]
              tunnel: w486 -> [_ w577]
              tunnel: w491 -> [_ w576]
              tunnel: w490 -> [_ w575]
              tunnel: [w572 w573] -> w485
              tunnel: w484 -> [w572 w574]
              frame False {
              }
              frame True {
                n184 = call "compute path cluster.vi"("path queue"=w577, "Arrive simultaeously"=w575, "error in (no error)"=w574, "Step length\n(IMAQ pixels)"=w576, "waypoint queue"=w578) -> ("error out"=w573:errorcluster)  [unwired: 2 in]
              }
            }
            n185 = case "Follow path" shown="True" w487 {
              tunnel: w486 -> [_ w522]
              tunnel: w485 -> [_ w523]
              tunnel: w483 -> [_ w525]
              tunnel: w482 -> [_ w524]
              tunnel: w480 -> [_ w521]
              tunnel: w479 -> [w494 w502]
              tunnel: [w494 w501] -> w478
              tunnel: [w493 w496] -> w477
              tunnel: w476 -> [w493 _]
              tunnel: w475 -> [_ w495]
              frame False {
              }
              frame True {
                w516 = TRUE ("Visible")
                n186 = local write "Display path"(FALSE ("Display path")) -> ()
                n187 = Flush Queue "Flush Waypts"(queue=w524, error in (no error)=w523) -> (error out=w515:errorcluster)  [unwired: 2 out]
                n188 = Get Queue Status(queue=w522, error in (no error)=w515) -> (queue out=w519:refnum<queue>, error out=w514:errorcluster, # elements in queue=w518:i32)  [unwired: 1 in, 5 out]
                n189 = property on="Pause" class="Bool (strict)"(error in=w514, "Visible"=w516) -> (error out=w513:errorcluster)  [unwired: 1 in, 1 out]
                n190 = property on="cancel path" class="Bool"(error in=w513, "Visible"=w516) -> (error out=w512:errorcluster)  [unwired: 1 in, 1 out]
                n191 = for {
                  N: w518 -> [_]
                  tunnel: w512 -> [w545]
                  tunnel: w525 -> [w547]
                  tunnel: w519 -> [w543]
                  tunnel: [w543] -> w517
                  tunnel: [FALSE ("Group traps")] -> w497
                  shift-right: [w534] -> w496
                  shift-left: _ -> [w536]
                  tunnel: [w533] -> w511
                  tunnel: [w530] -> w509 mode=indexing
                  tunnel: [w531] -> w505
                  tunnel: [TRUE ("Display path")] -> w503
                  tunnel: w495 -> [w526]
                  i -> [w531]
                  stop <- w540 stop-if-true
                  n192 = Dequeue Element(queue=w543, timeout in ms (-1)=0, error in (no error)=w545) -> (element=w535:T5, timed out?=w539:bool, error out=w546:errorcluster)  [unwired: 1 out]
                  n193 = while {
                    tunnel: [w564] -> w537
                    tunnel: ["cancel path"] -> w532
                    tunnel: w526 -> [w561]
                    stop <- w566 stop-if-true
                    n194 = local read "Stop program"() -> (w564:bool)
                    n195 = Wait (ms)(milliseconds to wait=w561) -> ()  [unwired: 1 out]
                    n196 = Or(x=w564, y="cancel path") -> (x .or. y?=w562:bool)
                    n197 = Implies(1:w562, 2:"Pause") -> (0:w566:bool)
                  }
                  n198 = case shown="True" "Skip step if \ntimed out" {
                    tunnel: w547 -> [w553 w558]
                    tunnel: w546 -> [w552 w556]
                    tunnel: [FALSE ("overflow?") w554] -> w538
                    tunnel: w535 -> [w551 w557]
                    tunnel: [w550 w555] -> w533
                    tunnel: 500 ("timeout in ms (-1)") -> [w549 _]
                    frame False {
                      n199 = Enqueue Element "Enqueue trap pos"(queue=w553, element=w551, timeout in ms (-1)=w549, error in (no error)=w552) -> (error out=w550:errorcluster)  [unwired: 2 out]
                    }
                    frame True {
                      n200 = Lossy Enqueue Element(queue=w558, element=w557, error in (no error)=w556) -> (overflow?=w554:bool, error out=w555:errorcluster)  [unwired: 2 out]
                    }
                  }
                  "Step \nskipped" <- w538
                  n201 = case shown="False" w537 {
                    tunnel: w536 -> [_ w560]
                    tunnel: w535 -> [w559 _]
                    tunnel: [w559 w560] -> w534
                    frame False {
                    }
                    frame True {
                    }
                  }
                  n202 = Or(x=w532, y=w537) -> (x .or. y?=w542:bool)
                  n203 = Or(x=w542, y=w539) -> (x .or. y?=w540:bool)
                  n204 = Tick Count (ms)() -> (millisecond timer value=w530:u32)
                }
                n205 = local read "Transpose SLM"() -> (w499:bool)
                n206 = call "Trap cluster 2 ROI.vi"("Switch X/Y"=w499, "Trap cluster"=w496, "ROI in"=w521) -> ("ROI out"=w520:T2)
                n207 = local write "Step \nskipped"(w497) -> ()
                n208 = local write "Create path"(w497) -> ()
                n209 = local write "Display path"(w503) -> ()
                n210 = local write "Group \nTraps"(w497) -> ()
                n211 = property on="Pause" class="Bool (strict)"(error in=w511, "Visible"=w497, "Value"=w497) -> (error out=w510:errorcluster)  [unwired: 1 in, 1 out]
                n212 = property on="cancel path" class="Bool"(error in=w510, "Visible"=w497) -> ()  [unwired: 1 in, 2 out]
                n213 = property on="follow path" class="Bool (strict)"("Value"=w497) -> ()  [unwired: 2 in, 2 out]
                n214 = property on="Monitor image" class="ImageControl"(error in=w502, "ROI"=w520) -> (error out=w501:errorcluster)  [unwired: 1 in, 1 out]
                n215 = Array Max & Min(array=w509) -> (max value=w508:u32, min value=w507:u32)  [unwired: 2 out]
                n216 = Subtract(x=w508, y=w507) -> (x-y=w506:u32)
                n217 = Increment(x=w505) -> (x+1=w500:i32)
                n218 = Divide(x=w506, y=w500) -> (x/y=→"Average step \ntime (ms)":dbl)
                n219 = Flush Queue "Flush Path"(queue=w517) -> ()  [unwired: 1 in, 3 out]
              }
            }
          }
        }
        n220 = First Call?() -> (First Call?: T/F=w339:bool)
        n221 = Or(x="Apply Corrections", y=w339) -> (x .or. y?=w340:bool)
        n222 = case shown="True" w340 {
          frame False {
          }
          frame True {
            n223 = call "Apply Corrections.vi"() -> ()  [unwired: 1 in]
          }
        }
      }
      frame True {
        n224 = property on="Cancel calibration" class="Bool"("Visible"=w581) -> ()  [unwired: 2 in, 2 out]
        n225 = flat-sequence {
          tunnel: [w606] -> w593
          tunnel: [w608] -> w592
          tunnel: w588 -> [w606]
          tunnel: [w598] -> w587
          tunnel: [w595] -> w586
          tunnel: w585 -> [w600]
          tunnel: [w599] -> w583
          tunnel: [w671] -> w591
          tunnel: w593 -> [w671]
          tunnel: w592 -> [w629]
          tunnel: [w667] -> w590
          tunnel: w589 -> [w670]
          tunnel: w587 -> [w669]
          tunnel: w586 -> [w666]
          tunnel: [w665] -> w584
          tunnel: w583 -> [w665]
          tunnel: [w627] -> w579
          tunnel: w591 -> [w736]
          tunnel: w584 -> [w734]
          tunnel: [w733] -> w582
          frame #0 {
            w609 = u32 8 items=["Zoom Tool"=8, "Selection Tool"=0, "Pan Tool"=9, "Point Tool"=1, "Line Tool"=2, "Rectangle Tool"=3, "Rotated Rectangle Tool"=12, "Polyline Tool"=10, "Polygon Tool"=5, "Freehand Tool"=11, "Closed Freehand Tool"=6, "Ellipse Tool"=4, "Annulus Tool"=7] ("Current ROI Tool")
            n226 = local read "Using monitoring camera\nfor measurements"() -> (w594:bool)
            n227 = local read "Coordinate mapping \n(IMAQ to SLM)"() -> (w595:T3)
            n228 = Bundle By Name(cluster=w595, "sX"=0.0, "sY"=0.0, "cX"=1.0 ("sX"), "cY"=1.0) -> (w598:T3)
            n229 = case shown="False" w594 {
              frame False {
                n230 = call <vilib>:"Application Directory.vi"() -> ("Application Directory"=w612:path)
                n231 = Build Path(base path=w612, name or relative path="Sub VIs\\Display Image.vi") -> (appended path=w615:path)
                n232 = Open VI Reference(vi path=w615) -> (vi reference=w614:refnum<vi>)  [unwired: 5 in, 1 out]
                n233 = property class="VI"(reference=w614, "Front Panel.Open"=TRUE ("Front Panel Window:Open")) -> ()  [unwired: 1 in, 2 out]
              }
              frame True {
              }
            }
            n234 = local write "Coordinate mapping \n(IMAQ to SLM)"(w598) -> ()
            n235 = property on="ok" class="Bool"("Visible"=TRUE ("ROI Tool Buttons Visibile:Zoom Tool Button Visible")) -> ()  [unwired: 2 in, 2 out]
            n236 = property on="Monitor image" class="ImageControl"("Current ROI Tool"=w609) -> ()  [unwired: 2 in, 2 out]
            n237 = call <vilib>:"Three Button Dialog.vi"("Center Button Text (\"No\")"="Manual" ("T button name (\"OK\")"), "Left Button Text (\"Yes\")"="Auto" ("F button name (\"Cancel\")"), "message"="Mark the center of the \ndisplayed spot using the \nzoom and the point tool, \nthen click the OK button. \n(Will be repeated three times)") -> ("Which Button?"=w608:T12)  [unwired: 8 in]
            n238 = property on="Monitor image" class="ImageControl"(error in=w600, "ROI"=T2 {"Global Rectangle"=[100, 100, 394, 354], "Contours"=[{"Contour Type"=0, "ROI Type"=1, "Points"=[100, 100]}]} ("ROI 2")) -> (error out=w599:errorcluster)  [unwired: 1 in, 1 out]
          }
          frame #1 {
            w623 = sgl 0.0 ("sX")
            w624 = sgl 1.0 ("cX")
            n239 = local read "Coordinate mapping \n(Monitor to Measurement)"() -> (w622:T3)
            n240 = for {
              tunnel: [w692] -> w660 mode=indexing
              tunnel: [w691] -> w659 mode=indexing
              tunnel: T5[] [{"X (IMAQ)"=[-85.0], "Y (IMAQ)"=[-85.0], "Z"=[0.0], "I"=[100.0], "Trap number"=[0], "ROI number"=[0], "Number of traps"=1, "Group"=[]}, {"X (IMAQ)"=[85.0], "Y (IMAQ)"=[-85.0], "Z"=[0.0], "I"=[100.0], "Trap number"=[0], "ROI number"=[0], "Number of traps"=1, "Group"=[]}, {"X (IMAQ)"=[-85.0], "Y (IMAQ)"=[85.0], "Z"=[0.0], "I"=[100.0], "Trap number"=[0], "ROI number"=[0], "Number of traps"=0, "Group"=[]}] -> [w690] mode=indexing
              tunnel: [w687] -> w647 mode=indexing
              tunnel: [w685] -> w646 mode=indexing
              tunnel: w670 -> [w689]
              tunnel: [w684] -> w635 mode=indexing
              tunnel: [w683] -> w634 mode=indexing
              tunnel: w629 -> [w682]
              tunnel: [w680] -> w628
              stop <- w681 stop-if-true
              n241 = Enqueue Element "Enqueue trap pos"(queue=w689, element=w690) -> ()  [unwired: 2 in, 3 out]
              n242 = case shown="\"Left Button\", Default" w682 {
                tunnel: [w697 w714 _ _] -> w692
                tunnel: [w696 w713 _ _] -> w691
                tunnel: [w693 w711 w724 w725] -> w681
                tunnel: [w695 w708 _ _] -> w684
                tunnel: [w694 w707 _ _] -> w683
                tunnel: [w693 w706 w724 w725] -> w680
                frame "Left Button", Default {
                  n243 = flat-sequence {
                    tunnel: [w705] -> w697
                    tunnel: [w704] -> w696
                    tunnel: [w703] -> w695
                    tunnel: [w702] -> w694
                    tunnel: [FALSE] -> w693
                    frame #0 {
                      n244 = Wait (ms)(milliseconds to wait=u32 300) -> ()  [unwired: 1 out]
                    }
                    frame #1 {
                      n245 = local read "Monitoring image"() -> (w701:T1)
                      n246 = local read "Measurement image"() -> (w700:T1)
                      n247 = call "Find spot in image.vi"("Image"=w701) -> ("Y Centroid"=w704:dbl, "X Centroid"=w705:dbl)  [unwired: 7 in]
                      n248 = call "Find spot in image.vi"("Image"=w700) -> ("Y Centroid"=w702:dbl, "X Centroid"=w703:dbl)  [unwired: 7 in]
                    }
                  }
                }
                frame "Center Button" {
                  n249 = while {
                    tunnel: [w722] -> w712
                    tunnel: [w719] -> w711
                    tunnel: [w717] -> w710
                    tunnel: [w716] -> w706
                    stop <- w720 stop-if-true
                    n250 = local read "Stop program"() -> (w716:bool)
                    n251 = global read "Global variables.vi" "Measurement ROI"() -> (w717:T13)
                    n252 = Wait (ms)(milliseconds to wait=u32 50) -> ()  [unwired: 1 out]
                    n253 = Or(x=w716, y="Cancel calibration") -> (x .or. y?=w719:bool)
                    n254 = property on="Monitor image" class="ImageControl"() -> ("ROI"=w722:T2)  [unwired: 2 in, 2 out]
                    n255 = Or(x="ok", y=w719) -> (x .or. y?=w720:bool)
                  }
                  n256 = Unbundle By Name(w710) -> ("Global Rectangle"=w709:i32[])  [unwired: 1 out]
                  n257 = Unbundle By Name(w712) -> ("Global Rectangle"=w715:i32[])  [unwired: 1 out]
                  n258 = Index Array(array=w715) -> (element #1=w714:i32, element #2=w713:i32)  [unwired: 2 in]
                  n259 = Index Array(array=w709) -> (element #1=w708:i32, element #2=w707:i32)  [unwired: 2 in]
                }
                frame "Right Button" {
                  w724 = TRUE
                }
                frame "Window Close" {
                  w725 = TRUE
                }
              }
              n260 = Unbundle By Name(w690) -> ("X (IMAQ)"=w688:sgl[], "Y (IMAQ)"=w686:sgl[])
              n261 = Index Array(array=w686) -> (element=w685:sgl)  [unwired: 1 in]
              n262 = Index Array(array=w688) -> (element=w687:sgl)  [unwired: 1 in]
            }
            n263 = Index Array(array=w659) -> (element #1=w661:dbl, element #2=w662:dbl)  [unwired: 2 in]
            n264 = Index Array(array=w660) -> (element #1=w663:dbl, element #2=w664:dbl)  [unwired: 2 in]
            n265 = Subtract(x=w664, y=w663) -> (x-y=w656:dbl)
            n266 = Subtract(x=w662, y=w661) -> (x-y=w654:dbl)
            n267 = Absolute Value(x=w654) -> (abs(x)=w653:dbl)
            n268 = Absolute Value(x=w656) -> (abs(x)=w655:dbl)
            n269 = Less?(x=w655, y=w653) -> (x < y?=w618:bool)
            n270 = case shown="False" w618 {
              tunnel: w660 -> [w677 w679]
              tunnel: w659 -> [w676 w678]
              tunnel: [w676 w679] -> w657
              tunnel: [w677 w678] -> w658
              frame False {
              }
              frame True {
              }
            }
            n271 = Index Array(array=w634) -> (element #1=w639:dbl, element #2=w638:dbl)  [unwired: 2 in]
            n272 = Index Array(array=w635) -> (element #1=w637:dbl, element #2=w636:dbl)  [unwired: 2 in]
            n273 = Subtract(x=w636, y=w637) -> (x-y=w640:dbl)
            n274 = Subtract(x=w638, y=w639) -> (x-y=w642:dbl)
            n275 = Absolute Value(x=w642) -> (abs(x)=w643:dbl)
            n276 = Absolute Value(x=w640) -> (abs(x)=w641:dbl)
            n277 = Less?(x=w641, y=w643) -> (x < y?=w619:bool)
            n278 = case shown="False" w619 {
              tunnel: w635 -> [w673 w675]
              tunnel: w634 -> [w672 w674]
              tunnel: [w672 w675] -> w644
              tunnel: [w673 w674] -> w645
              frame False {
              }
              frame True {
              }
            }
            n279 = formula code="cX = (xSLM[1] - xSLM[0]) / (xMonitor[1] - xMonitor[0]); \ncY = (ySLM[2] - ySLM[0]) / (yMonitor[2] - yMonitor[0]); \n\nsX = xSLM[0] - xMonitor[0] *cX;\nsY = ySLM[0] - yMonitor[0] *cY;\n\ncXm = (xMeasure[1] - xMeasure[0]) / (xMonitor[1] - xMonitor[0]); \ncYm = (yMeasure[2] - yMeasure[0]) / (yMonitor[2] - yMonitor[0]); \n\nsXm = xMeasure[0] - xMonitor[0] *cXm;\nsYm = yMeasure[0] - yMonitor[0] *cYm;"("xMonitor"=w658, "yMonitor"=w657, "xSLM"=w647, "ySLM"=w646, "xMeasure"=w645, "yMeasure"=w644) -> ("cX"=w652:dbl, "cY"=w651:dbl, "sX"=w650:dbl, "sY"=w649:dbl, "cXm"=w633:dbl, "cYm"=w632:dbl, "sXm"=w631:dbl, "sYm"=w630:dbl)
            n280 = local read "Using monitoring camera\nfor measurements"() -> (w617:bool)
            n281 = Select(t=FALSE, s=w617, f=w619) -> (s? t:f=w620:bool)
            n282 = Bundle By Name(cluster=w669, "cX"=w652, "cY"=w651, "sX"=w650, "sY"=w649) -> (w668:T3)
            n283 = Bundle By Name(cluster=w622, "cX"=w624, "cY"=w624, "sX"=w623, "sY"=w623) -> (w621:T3)
            n284 = Bundle By Name(cluster=w622, "cX"=w633, "cY"=w632, "sX"=w631, "sY"=w630) -> (w625:T3)
            n285 = Select(t=w621, s=w617, f=w625) -> (s? t:f=w626:T3)
            n286 = case "Calibration canceled?" shown="False" w628 {
              tunnel: w668 -> [w729 _]
              tunnel: [w729 w731] -> w667
              tunnel: w666 -> [_ w731]
              tunnel: [w726 w730] -> w627
              tunnel: w626 -> [w726 w730]
              tunnel: w620 -> [w728 _]
              tunnel: w618 -> [w727 _]
              frame False {
                n287 = local write "Transpose Measurement"(w728) -> ()
                n288 = local write "Transpose SLM"(w727) -> ()
              }
              frame True {
              }
            }
          }
          frame #2 {
            w732 = FALSE ("ROI Tool Buttons Visibile:Zoom Tool Button Visible")
            w735 = u32 1 items=["Zoom Tool"=8, "Selection Tool"=0, "Pan Tool"=9, "Point Tool"=1, "Line Tool"=2, "Rectangle Tool"=3, "Rotated Rectangle Tool"=12, "Polyline Tool"=10, "Polygon Tool"=5, "Freehand Tool"=11, "Closed Freehand Tool"=6, "Ellipse Tool"=4, "Annulus Tool"=7] ("Current ROI Tool")
            n289 = property on="Monitor image" class="ImageControl"(error in=w734, "ROI"=w736) -> (error out=w733:errorcluster)  [unwired: 1 in, 1 out]
            n290 = property on="Monitor image" class="ImageControl"("Current ROI Tool"=w735, "Point Tool Button Visibile"=w732) -> ()  [unwired: 2 in, 2 out]
            n291 = property on="Cancel" class="Bool"("Visible"=w732) -> ()  [unwired: 2 in, 2 out]
            n292 = property on="ok" class="Bool"("Visible"=w732) -> ()  [unwired: 2 in, 2 out]
          }
        }
        n293 = local write "Coordinate mapping \n(IMAQ to SLM)"(w590) -> ()
        n294 = local write "Coordinate mapping \n(Monitor to Measurement)"(w579) -> ()
      }
    }
  }
  n295 = while "User input and events loop" {
    tunnel: w79 -> [w757]
    tunnel: w25 -> [w746]
    tunnel: w57 -> [w745]
    tunnel: w24 -> [w744]
    tunnel: [w743] -> w66
    tunnel: w65 -> [w742]
    tunnel: [w741] -> w64
    tunnel: w47 -> [w739]
    tunnel: w2 -> [w738]
    tunnel: w10 -> [w737]
    stop <- w749 stop-if-true
    w754 = u32 8 items=["Zoom Tool"=8, "Selection Tool"=0, "Pan Tool"=9, "Point Tool"=1, "Line Tool"=2, "Rectangle Tool"=3, "Rotated Rectangle Tool"=12, "Polyline Tool"=10, "Polygon Tool"=5, "Freehand Tool"=11, "Closed Freehand Tool"=6, "Ellipse Tool"=4, "Annulus Tool"=7] ("Current ROI Tool")
    w751 = T14 [enum."LCONTROL"] items=["0", "1", "2", "3", "4", "5", "6", "7", "8", "9", "A", "B", "C", "D", "E", "F", "G", "H", "I", "J", "K", "L", "M", "N", "O", "P", "Q", "R", "S", "T", "U", "V", "W", "X", "Y", "Z", "F1", "F2", "F3", "F4", "F5", "F6", "F7", "F8", "F9", "F10", "F11", "F12", "F13", "F14", "F15", "ADD", "BACK", "BACKSLASH", "CAPITAL", "COMMA", "DECIMAL", "DELETE", "DIVIDE", "DOWN", "END", "EQUALS", "ESCAPE", "GRAVE (`)", "HOME", "INSERT", "LBRACKET", "LCONTROL", "LEFT", "L ALT", "LSHIFT", "LWIN", "MINUS", "MULTIPLY", "NEXT", "NUMLOCK", "NUMPAD_0", "NUMPAD_1", "NUMPAD_2", "NUMPAD_3", "NUMPAD_4", "NUMPAD_5", "NUMPAD_6", "NUMPAD_7", "NUMPAD_8", "NUMPAD_9", "PAUSE", "PERIOD", "PRIOR (PG UP)", "RBRACKET", "RCONTROL", "RETURN", "RIGHT", "R ALT", "RSHIFT", "RWIN", "SCROLL", "SEMICOLON", "SLASH", "SPACE", "SUBTRACT", "TAB", "UP", "ENTER (num pad)", "' (quote)"] ("keys pressed")
    n296 = call-poly <vilib>:"Acquire Input Data.vi"("device ID"=w757, "error in (no error)"=w742) -> ("device ID"=w743:refnum<k1>, "keys pressed"=w750:T14, "error out"=w741:errorcluster)  [unwired: 15 out]
    n297 = property on="Monitor image" class="ImageControl"() -> ("Current ROI Tool"=w753:u32)  [unwired: 2 in, 2 out]
    n298 = Equal?(x=w750, y=w751) -> (x = y?=w752:bool[])
    n299 = Not Equal?(x=w753, y=w754) -> (x != y?=w755:bool)
    n300 = Or Array Elements(Boolean array=w752) -> (logical OR=w756:bool)
    n301 = case shown="True" w755 {
      tunnel: w756 -> [_ w852]
      frame False {
      }
      frame True {
        n302 = case shown="False" w852 {
          frame False {
            w853 = u32 0 items=["Zoom Tool"=8, "Selection Tool"=0, "Pan Tool"=9, "Point Tool"=1, "Line Tool"=2, "Rectangle Tool"=3, "Rotated Rectangle Tool"=12, "Polyline Tool"=10, "Polygon Tool"=5, "Freehand Tool"=11, "Closed Freehand Tool"=6, "Ellipse Tool"=4, "Annulus Tool"=7] ("Current ROI Tool")
            n303 = property on="Monitor image" class="ImageControl"("Current ROI Tool"=w853) -> ()  [unwired: 2 in, 2 out]
          }
          frame True {
            w854 = u32 1 items=["Zoom Tool"=8, "Selection Tool"=0, "Pan Tool"=9, "Point Tool"=1, "Line Tool"=2, "Rectangle Tool"=3, "Rotated Rectangle Tool"=12, "Polyline Tool"=10, "Polygon Tool"=5, "Freehand Tool"=11, "Closed Freehand Tool"=6, "Ellipse Tool"=4, "Annulus Tool"=7] ("Current ROI Tool")
            n304 = property on="Monitor image" class="ImageControl"("Current ROI Tool"=w854) -> ()  [unwired: 2 in, 2 out]
          }
        }
      }
    }
    n305 = Wait (ms)(milliseconds to wait=u32 50) -> ()  [unwired: 1 out]
    n306 = case shown="False" "View Licence" {
      frame False {
      }
      frame True {
        n307 = call "View license.vi"() -> ()  [unwired: 1 in]
      }
    }
    n308 = event shown="[1] \"Display hologram and computed  image plane\": Value Change" {
      selector: _ -> [_ _ _ _ _ _ _ _ _ _ _ _ _ _]
      dyn-events: _ -> [_ _ _ _ _ _ _ _ _ _ _ _ _ _]
      timeout: 0 -> [_ _ _ _ _ _ _ _ _ _ _ _ _ _]
      tunnel: w746 -> [_ _ w764 _ _ _ _ _ _ _ _ _ _ _]
      tunnel: w745 -> [_ _ w763 _ _ _ _ _ _ _ _ _ _ _]
      tunnel: w744 -> [_ _ w767 _ _ _ _ _ _ _ _ _ _ _]
      tunnel: w739 -> [_ _ _ _ _ _ w780 _ _ _ _ _ _ _]
      tunnel: w738 -> [_ _ _ _ _ _ _ _ _ _ _ w800 w824 w845]
      tunnel: w737 -> [_ _ _ _ _ _ _ _ _ _ _ w799 w823 w843]
      tunnel: [_ _ _ _ _ _ _ _ _ _ _ _ w822 _] -> _
      tunnel: [_ _ _ _ _ _ _ _ _ _ _ _ w821 _] -> _
      event Timeout {
        n309 = event-data() -> ()  [unwired: 1 in, 2 out]
      }
      event "Display hologram\nand computed \nimage plane": Value Change {
        n310 = event-data() -> ("NewVal"=w758:bool)  [unwired: 1 in, 4 out]
        n311 = property on="Current trap pos" class="Clust (strict)"("Visible"=w758) -> ()  [unwired: 2 in, 2 out]
        n312 = call <vilib>:"Application Directory.vi"() -> ("Application Directory"=w759:path)
        n313 = Build Path(base path=w759, name or relative path="Sub VIs\\Calculate farfield intensity.vi") -> (appended path=w762:path)
        n314 = Open VI Reference(vi path=w762) -> (vi reference=w761:refnum<vi>)  [unwired: 5 in, 1 out]
        n315 = property class="VI"(reference=w761, "Front Panel.Open"=w758) -> ()  [unwired: 1 in, 2 out]
      }
      event "Create path": Value Change {
        n316 = event-data() -> ()  [unwired: 1 in, 5 out]
        n317 = property on="follow path" class="Bool (strict)"("Value"=FALSE) -> ()  [unwired: 2 in, 2 out]
        n318 = Flush Queue "Flush path \nwaypt queue"(queue=w763) -> ()  [unwired: 1 in, 3 out]
        n319 = Preview Queue Element(queue=w764) -> (element=w765:T5, error out=w768:errorcluster)  [unwired: 2 in, 2 out]
        n320 = Flush Queue "Flush path queue"(queue=w767) -> (queue out=w766:refnum<queue>)  [unwired: 1 in, 2 out]
        n321 = Enqueue Element "Enqueue current \ntrap pos in path"(queue=w766, element=w765) -> ()  [unwired: 2 in, 3 out]
        n322 = Enqueue Element "Enqueue current \ntrap pos in path \nwaypts"(queue=w763, element=w765, error in (no error)=w768) -> ()  [unwired: 1 in, 3 out]
      }
      event "cancel path": Value Change {
        n323 = event-data() -> ()  [unwired: 1 in, 5 out]
        n324 = local write "Create path"(FALSE ("Visible")) -> ()
      }
      event "Monitor image", "Group \nTraps", "Z", "I", "Coordinate mapping \n(IMAQ to SLM)": Mouse Down {
        w771 = FALSE ("Edit trap cluster")
        n325 = event-data() -> ()  [unwired: 1 in, 7 out]
        n326 = local write "Updating trap cluster"(TRUE ("Update trap positions")) -> ()
        n327 = local write "Edit trap cluster"(w771) -> ()
        n328 = call <vilib>:"Application Directory.vi"() -> ("Application Directory"=w772:path)
        n329 = Build Path(base path=w772, name or relative path="Sub VIs\\Edit trap cluster.vi") -> (appended path=w775:path)
        n330 = Open VI Reference(vi path=w775) -> (vi reference=w774:refnum<vi>)  [unwired: 5 in, 1 out]
        n331 = property class="VI"(reference=w774, "Front Panel.Open"=w771) -> ()  [unwired: 1 in, 2 out]
      }
      event "Group \nTraps", "Z", "I", "Monitor image", "Coordinate mapping \n(IMAQ to SLM)": Mouse Up {
        n332 = event-data() -> ()  [unwired: 1 in, 7 out]
        n333 = flat-sequence {
          frame #0 {
            n334 = Wait (ms)(milliseconds to wait=u32 100) -> ()  [unwired: 1 out]
          }
          frame #1 {
            n335 = local write "Updating trap cluster"(FALSE ("Update trap positions")) -> ()
          }
        }
      }
      event "Record": Value Change {
        n336 = event-data() -> ()  [unwired: 1 in, 5 out]
        n337 = Unbundle By Name(w780) -> ("Image buffers"=w779:T1[])
        n338 = for {
          tunnel: w779 -> [w781] mode=indexing
          n339 = call "IMAQ Clear Overlay"("Image"=w781) -> ()  [unwired: 9 in, 2 out]
        }
      }
      event "Display data": Value Change {
        n340 = event-data() -> ("NewVal"=w783:bool)  [unwired: 1 in, 4 out]
        n341 = call <vilib>:"Application Directory.vi"() -> ("Application Directory"=w782:path)
        n342 = Build Path(base path=w782, name or relative path="Sub VIs\\Display Cetroids (SubVI).vi") -> (appended path=w786:path)
        n343 = Open VI Reference(vi path=w786) -> (vi reference=w785:refnum<vi>)  [unwired: 5 in, 1 out]
        n344 = property class="VI"(reference=w785, "Front Panel.Open"=w783) -> ()  [unwired: 1 in, 2 out]
      }
      event "Display ROIs": Value Change {
        n345 = event-data() -> ("NewVal"=w787:bool)  [unwired: 1 in, 4 out]
        n346 = call <vilib>:"Application Directory.vi"() -> ("Application Directory"=w788:path)
        n347 = Build Path(base path=w788, name or relative path="Sub VIs\\Display ROIs.vi") -> (appended path=w791:path)
        n348 = Open VI Reference(vi path=w791) -> (vi reference=w790:refnum<vi>)  [unwired: 5 in, 1 out]
        n349 = property class="VI"(reference=w790, "Front Panel.Open"=w787) -> ()  [unwired: 1 in, 2 out]
      }
      event "Display ROIs": Value Change {
        n350 = event-data() -> ("NewVal"=w792:bool)  [unwired: 1 in, 4 out]
        n351 = call <vilib>:"Application Directory.vi"() -> ("Application Directory"=w793:path)
        n352 = Build Path(base path=w793, name or relative path="Sub VIs\\Display Image.vi") -> (appended path=w796:path)
        n353 = Open VI Reference(vi path=w796) -> (vi reference=w795:refnum<vi>)  [unwired: 5 in, 1 out]
        n354 = property class="VI"(reference=w795, "Front Panel.Open"=w792) -> ()  [unwired: 1 in, 2 out]
      }
      event "Edit trap cluster": Value Change {
        n355 = event-data() -> ("NewVal"=w797:bool)  [unwired: 1 in, 4 out]
        n356 = local write "Updating trap cluster"(w797) -> ()
      }
      event "Save data": Value Change {
        n357 = event-data() -> ()  [unwired: 1 in, 5 out]
        n358 = Flush Queue(queue=w800) -> (remaining elements=w810:T15)  [unwired: 1 in, 2 out]
        n359 = Flush Queue(queue=w799) -> (remaining elements=w805:T5[])  [unwired: 1 in, 2 out]
        n360 = for {
          tunnel: [w820] -> w813 mode=indexing
          tunnel: [w819] -> w812 mode=indexing
          tunnel: [w818] -> w806 mode=indexing
          tunnel: w810 -> [w817] mode=indexing
          tunnel: w805 -> [w816] mode=indexing
          tunnel: [w815] -> w804 mode=indexing
          tunnel: [w814] -> w803 mode=indexing
          n361 = Unbundle By Name(w817) -> ("CentroidX"=w820:dbl[], "CentroidY"=w819:dbl[], "Acquired Buffer Number"=w818:u32)
          n362 = Unbundle By Name(w816) -> ("X (IMAQ)"=w815:sgl[], "Y (IMAQ)"=w814:sgl[])
        }
        n363 = Transpose 2D Array(2D array=w813) -> (transposed array=w809:dbl[][])
        n364 = Transpose 2D Array(2D array=w812) -> (transposed array=w808:dbl[][])
        n365 = Transpose 2D Array(2D array=w804) -> (transposed array=w802:sgl[][])
        n366 = Transpose 2D Array(2D array=w803) -> (transposed array=w801:sgl[][])
        n367 = Build Array (concatenate)(w806, w809, w808, w802, w801) -> (w798:dbl[][])
        n368 = Transpose 2D Array(2D array=w798) -> (transposed array=w807:dbl[][])
        n369 = call-poly <vilib>:"Write To Spreadsheet File.vi"("format (%.3f)"="%.9f", "2D data"=w807) -> ()  [unwired: 6 in, 1 out]
      }
      event "Purge data": Value Change {
        n370 = event-data() -> ()  [unwired: 1 in, 5 out]
        n371 = Flush Queue(queue=w824) -> (remaining elements=w822:T15)  [unwired: 1 in, 2 out]
        n372 = Flush Queue(queue=w823) -> (remaining elements=w821:T5[])  [unwired: 1 in, 2 out]
      }
      event "Run meas calibration": Value Change {
        w842 = TRUE ("return elements? (F)")
        n373 = event-data() -> ()  [unwired: 1 in, 5 out]
        n374 = local read "Coordinate mapping \n(Monitor to Measurement)"() -> (w827:T3)
        n375 = Get Queue Status(queue=w845, return elements? (F)=w842) -> (elements=w844:T15)  [unwired: 1 in, 7 out]
        n376 = Get Queue Status(queue=w843, return elements? (F)=w842) -> (elements=w841:T5[])  [unwired: 1 in, 7 out]
        n377 = for {
          tunnel: w844 -> [w851] mode=indexing
          tunnel: w841 -> [_] mode=indexing
          tunnel: w841 -> [w850] mode=indexing
          tunnel: [w849] -> w834 mode=indexing
          tunnel: [w848] -> w838 mode=indexing
          tunnel: [w847] -> w833 mode=indexing
          tunnel: [w846] -> w831 mode=indexing
          n378 = Unbundle By Name(w851) -> ("CentroidX"=w848:dbl[], "CentroidY"=w847:dbl[])
          n379 = Unbundle By Name(w850) -> ("X (IMAQ)"=w849:sgl[], "Y (IMAQ)"=w846:sgl[])
        }
        n380 = Array Size(array=w834) -> (size(s)=w839:i32[])
        n381 = Multiply Array Elements(1:w839) -> (0:w825:i32)
        n382 = Reshape Array(w831, w825) -> (w830:sgl[])
        n383 = Reshape Array(w833, w825) -> (w832:dbl[])
        n384 = Reshape Array(w834, w825) -> (w840:sgl[])
        n385 = Reshape Array(w838, w825) -> (w837:dbl[])
        n386 = call <vilib>:"Linear Fit.vi"("Y"=w837, "X"=w840) -> ("slope"=w836:dbl, "intercept"=w835:dbl)  [unwired: 9 in, 3 out]
        n387 = call <vilib>:"Linear Fit.vi"("Y"=w832, "X"=w830) -> ("slope"=w829:dbl, "intercept"=w828:dbl)  [unwired: 9 in, 3 out]
        n388 = Bundle By Name(cluster=w827, "cX"=w836, "sX"=w835, "cY"=w829, "sY"=w828) -> (w826:T3)
        n389 = local write "Coordinate mapping \n(Monitor to Measurement)"(w826) -> ()
      }
    }
    n390 = local read "Stop program"() -> (w749:bool)
  }
  n391 = Unbundle By Name(w37) -> ("Camera type"=w29:T8)
  n392 = local read "Using monitoring camera\nfor measurements"() -> (w28:bool)
  n393 = call "IMAQ Create"("Image Name"="Monitoring copy", "Image Type"=w19) -> ("New Image"=w26:T1)  [unwired: 3 in, 1 out]
  n394 = while {
    tunnel: w37 -> [w872]
    tunnel: [w870] -> w30
    tunnel: w29 -> [w871]
    tunnel: w28 -> [w868]
    tunnel: w26 -> [w867]
    tunnel: w25 -> [w866]
    tunnel: w24 -> [w860]
    tunnel: w23 -> [w855]
    stop <- w873 stop-if-true
    n395 = Preview Queue Element(queue=w866, timeout in ms (-1)=10) -> (element=w865:T5)  [unwired: 1 in, 3 out]
    n396 = case shown="False" w868 {
      tunnel: w872 -> [w878 w881]
      tunnel: w871 -> [w877 _]
      tunnel: [w876 w882] -> w864
      tunnel: [w875 w879] -> w870
      tunnel: w867 -> [_ w884]
      frame False {
        n397 = call "Acquire image (SubVI).vi"("Camera type"=w877, "Measurement camera \ncluster in"=w878) -> ("Image Out"=w876:T1, "Measurement camera cluster out"=w875:T10)  [unwired: 7 in, 1 out]
      }
      frame True {
        n398 = Unbundle By Name(w881) -> ("Image"=w885:T1, "Camera error"=w883:errorcluster)
        n399 = call "IMAQ Copy"("error in (no error)"=w883, "Image Dst"=w884, "Image Src"=w885) -> ("error out"=w880:errorcluster, "Image Dst Out"=w882:T1)  [unwired: 3 in]
        n400 = Bundle By Name(cluster=w881, "Camera error"=w880) -> (w879:T10)
      }
    }
    n401 = Wait (ms)(milliseconds to wait=u32 200) -> ()  [unwired: 1 out]
    n402 = local read "Stop program"() -> (w873:bool)
    n403 = local read "ROI \nsize"() -> (w863:dbl)
    n404 = Get Queue Status(queue=w860, return elements? (F)="Display path") -> (elements=w861:T5[])  [unwired: 1 in, 7 out]
    n405 = local read "Transpose SLM"() -> (w862:bool)
    n406 = case shown="False" "Display ROIs" {
      tunnel: w855 -> [_ w874]
      frame False {
      }
      frame True {
        n407 = call "Display ROIs.vi"("ROI array in"=w874) -> ()  [unwired: 11 in]
      }
    }
    n408 = call "Create trap overlay.vi"("Current trap cluster"=w865, "Image in"=w864, "ROI size"=w863, "Switch X/Y"=w862, "Path"=w861) -> ("Image Out"=→"Monitor image":T1)
  }
  n409 = Unbundle By Name(w30) -> ("Camera type"=w36:T8, "IMAQ Session"=w35:refnum<k11>, "IMAQdx Session"=w34:T9, "Camera error"=w33:errorcluster, "Image"=w32:T1, "Image buffers"=w31:T1[])
  n410 = case shown="\"IMAQdx (firewire)\"" w36 {
    tunnel: w35 -> [w889 _ _ w898]
    tunnel: [w888 w893 w894 w897] -> _
    tunnel: w34 -> [_ w892 _ _]
    tunnel: w33 -> [w887 w891 w894 w896]
    tunnel: w32 -> [w886 w890 _ _]
    tunnel: w31 -> [_ _ _ w895]
    frame "IMAQ (Camera Link)", Default {
      n411 = call <vilib>:"IMAQ Close.vi"("error in (no error)"=w887, "IMAQ Session In"=w889) -> ("error out"=w888:errorcluster)  [unwired: 9 in]
      n412 = call "IMAQ Dispose"("Image"=w886) -> ()  [unwired: 5 in, 1 out]
    }
    frame "IMAQdx (firewire)" {
      n413 = call <vilib>:"IMAQdx Close Camera.vi"("error in"=w891, "Session In"=w892) -> ("error out"=w893:errorcluster)  [unwired: 9 in]
      n414 = call "IMAQ Dispose"("Image"=w890) -> ()  [unwired: 5 in, 1 out]
    }
    frame "No camera" {
    }
    frame "IMAQ ring" {
      n415 = call <vilib>:"IMAQ Close.vi"("error in (no error)"=w896, "IMAQ Session In"=w898) -> ("error out"=w897:errorcluster)  [unwired: 9 in]
      n416 = for {
        tunnel: w895 -> [w899] mode=indexing
        n417 = call "IMAQ Dispose"("Image"=w899) -> ()  [unwired: 5 in, 1 out]
      }
    }
  }
  n418 = call "FreeGPUandSLM.vi"("error in"=w46) -> ("error out"=w68:errorcluster)  [unwired: 1 out]
  "CUDA/SLM error" <- w68
  n419 = Unbundle By Name(w40) -> ("Camera type"=w44:T8, "IMAQ Session"=w43:refnum<k11>, "IMAQdx Session"=w42:T9, "Camera error"=w41:errorcluster, "Image"=w39:T1, "Image buffers"=w38:T1[])
  n420 = case shown="\"IMAQ ring\"" w44 {
    tunnel: w43 -> [w903 _ _ w912]
    tunnel: [w902 w907 w908 w911] -> w70
    tunnel: w42 -> [_ w906 _ _]
    tunnel: w41 -> [w901 w905 w908 w910]
    tunnel: w39 -> [w900 w904 _ _]
    tunnel: w38 -> [_ _ _ w909]
    frame "IMAQ (Camera Link)", Default {
      n421 = call <vilib>:"IMAQ Close.vi"("error in (no error)"=w901, "IMAQ Session In"=w903) -> ("error out"=w902:errorcluster)  [unwired: 9 in]
      n422 = call "IMAQ Dispose"("Image"=w900) -> ()  [unwired: 5 in, 1 out]
    }
    frame "IMAQdx (firewire)" {
      n423 = call <vilib>:"IMAQdx Close Camera.vi"("error in"=w905, "Session In"=w906) -> ("error out"=w907:errorcluster)  [unwired: 9 in]
      n424 = call "IMAQ Dispose"("Image"=w904) -> ()  [unwired: 5 in, 1 out]
    }
    frame "No camera" {
    }
    frame "IMAQ ring" {
      n425 = for {
        tunnel: w909 -> [w913] mode=indexing
        n426 = call "IMAQ Dispose"("Image"=w913) -> ()  [unwired: 5 in, 1 out]
      }
      n427 = call <vilib>:"IMAQ Close.vi"("error in (no error)"=w910, "IMAQ Session In"=w912) -> ("error out"=w911:errorcluster)  [unwired: 9 in]
    }
  }
  n428 = call-poly <vilib>:"Close Input Device.vi"("error in (no error)"=w64, "device ID"=w66) -> ()  [unwired: 9 out]
  n429 = Unbundle By Name(w71) -> ("Contours"=w76:T16)
  n430 = Index Array(array=w76) -> (element=w75:T17)  [unwired: 1 in]
  n431 = Merge Errors(w70, w69) -> (w67:errorcluster)
  "NI Vision error" <- w67
  n432 = flat-sequence {
    tunnel: w68 -> [_]
    tunnel: w67 -> [_]
    frame #0 {
      n433 = local write "Stop program"(FALSE ("Stop program")) -> ()
    }
  }
  n434 = Unbundle By Name(w75) -> ("ROI Type"=w74:u32)
  n435 = Equal?(x=w74, y=u32 1) -> (x = y?=w72:bool)
  n436 = case shown="True" w72 {
    tunnel: w71 -> [_ w915]
    frame False {
    }
    frame True {
      n437 = local write "ROI"(w915) -> ()
    }
  }
